vi "UHR-Fleezers Control (fpga) - 11.7.1UCBMeng3RG2.vi"() -> ()   [LabVIEW 2014]
doc: "UHR-Fleezers Instrument Control Code (fpga)"
uses:
  <vilib>/Platform/TimedLoop/XDataNode/timing_clust.ctl
  <vilib>/Platform/TimedLoop/XDataNode/nitl_modes.ctl
  <vilib>/Platform/TimedLoop/XDataNode/wakeup.ctl
  <vilib>/rvi/Emulation/niFpgaGetClockAttributes.vi
  <vilib>/rvi/Emulation/niFpgaSctlEmulationGetInTimedLoop.vi
  <vilib>/rvi/Emulation/niFpgaEmulationReportErrorSimple.vi
  <vilib>/rvi/Emulation/niFpgaProcessEmulError.vi
  <vilib>/rvi/eio/common/nirviEmuTemplateMethod_errors.vi
  <vilib>/rvi/Emulation/niFpgaCriticalErrorInLSC.vi
  <vilib>/rvi/interface/RandomDataEmulation/niFpgaRandomDataHandleErrors.vi
  <vilib>/eio/EIONode/EIONode.xnode
  <vilib>/eio/EIOMethodNode/EIOMethodNode.xnode
  <vilib>/rvi/DataTransferAndStorage/Container/XNode/niFpgaContainer.xnode
  <vilib>/rvi/interface/RandomDataEmulation/nirviRandomDataFpgaReadWriteTemplate.vi
  <vilib>/addons/control/pid/fpga.llb/XNode/niFpgaPID.xnode
  <vilib>/Platform/TimedLoop/XDataNode/XDataNode.xnode
  <vilib>/Platform/TimedLoop/XDataNode/XDNodeRunTimeDep.lvlib
panel:
  in  "Tab Control":T1(tab)=enum."Force FB"
  in  "Set 3":bool
  in  "Set 2":bool=TRUE
  in  "Set 1":bool=TRUE
  in  "Trap Pos to FIFO":bool
  in  "N of AI1 Int Acq Sets":i16=2 min=1 max=3 step=1
  out "AI Late Counter":u8
  in  "ai count":u16=400
  in  "+ phase":bool
  in  "Phase count adjustment":i16
  out "Relative phase":i16
  in  "AI to FIFO":bool
  out "BD1 Frequency Out 1":u64
  out "BD1 Frequency Out 2":u64
  out "Trap Pos FIFO Timeout":u16
  out "Trap AI FIFO Timeout":u16
  in  "Trap FIFO Set Timeout":i32
  in  "Tab Control 2":T2(tab)
  in  "FB Offset":u16
  in  "FB Multi Factor":i16
  in  "Dynamic FB (Ronen)":bool
  in  "Negate Intensity FB":bool
  in  "RD":bool
  in  "FB1 output high":i16=3000
  in  "FB1 output low":i16
  in  "D1":i16
  in  "I1":i16=5
  in  "P1":i16=10
  in  "Swap F1 and F2":bool
  in  "Cont. Scan":bool
  in  "Abort scan":bool
  in  "Cycles per step":u64
  in  "Scan BD":bool
  in  "Number of scans":u16
  in  "Scan steps":u64
  in  "Scan freq.  increment":i64
  out "Scanning":bool
  in  "Start scan":bool
  in  "OSK Bd 1":bool
  in  "Reset Bd 1":bool
  in  "PMODE":bool
  in  "Direct RF Box \nCommunication":bool
  in  "Data BD 2":u8 format="%08b"
  in  "Data BD 1":u8 format="%08b"
  in  "Address":u8 format="%02x"
  in  "Update Data":bool
  in  "FPGA Controls\n RF Box":bool
  in  "Number Interlace Cycles":u8=2 min=1 max=3
  in  "Interlace Off Parameters":u8=1 min=1 max=3
  in  "Interlace ON/OFF":bool
  out "DIO Relative phase":i16
  in  "Phase count adjustment (DIO)":i16
  in  "+ phase (DIO)":bool
  out "DIO Late Counter":u8
  in  "DIO count 1 (ticks)":u16=400
  in  "DIO count 2 (ticks)":u16=400
  in  "DIO count 3 (ticks)":u16=400
  out "AI2 Y Sum Set 2":i16
  out "AI2 Y Sum Set 1":i16
  in  "FB Setpoint Set 1":i16 min=0 step=1
  in  "FB Reset Set 1":bool
  in  "FB On/Off Set 1":bool
  in  "FB Reset Set 2":bool
  in  "FB On/Off Set 2":bool
  in  "FB Setpoint Set 2":i16 min=0 step=1
  out "Scan I":u64
  in  "Amp switch delay":u8=5
  in  "XY phase ext loop method":bool
  in  "BD 2 Amplitude 1":u16
  in  "BD 1 Amplitude 1":u16
  in  "BD 2 Frequency 1":u64
  in  "BD 1 Frequency 1":u64
  in  "BD 2 Amplitude 2":u16
  in  "BD 1 Amplitude 2":u16
  in  "BD 2 Frequency 2":u64
  in  "BD 1 Frequency 2":u64
  in  "BD 2 Amplitude 3":u16
  in  "BD 1 Amplitude 3":u16
  in  "BD 2 Frequency 3":u64
  in  "BD 1 Frequency 3":u64
  in  "BD 1 Delay (ticks)":u8
  in  "BD 2 Delay (Ticks)":u8 caption="Count(Ticks)"
  in  "Next trap write delay (ticks)":u8 caption="Count(Ticks)"
  in  "Trap 1 osc enable":bool
  in  "Trap 2 osc enable":bool
  in  "Dynamic Force FB (Ronen)":bool
  in  "FB2 output high":fxp<+/-,16,1>=0.999969482421875
  in  "FB2 output low":fxp<+/-,16,1>=-1.0
  in  "P2":fxp<+/-,16,8> format="%.11g"
  in  "I2":fxp<+/-,16,8>=10.0 format="%.11g"
  in  "D2":fxp<+/-,16,8> format="%.11g"
  in  "Negate Diff?":bool
  in  "Diff FB Measurement?":bool
  in  "FB Trig Integrate":u32=1
  out "TTrig?":bool
  in  "TTrig Negate Pos":bool=TRUE
  out "Trap Pos FB Int Signal":fxp<+/-,24,9> format="%.18g"
  out "Trap Pos FB Int-Norm Signal":fxp<+/-,16,1> format="%.16g"
  in  "FPGA TTrig Thresh":i64
  in  "FPGA Trap Trig":bool
  out "Trap Pos FB Action":i64
  in  "Trap Pos. FB Offset Factor":i64
  in  "Trap Pos. FB Mult Factor":i64=2
  in  "Trap Pos. FB Reset":bool
  in  "Trap Pos FB Monitor T1 or T2":bool
  in  "AI1 X Scale":u16
  in  "Trap Pos FB Int Count":u16=100
  in  "Trap Pos FB Negate Action":bool
  out "AI1 X Set 2":fxp<+/-,16,1>
  out "AI1 X Set 1":fxp<+/-,16,1>
  in  "Trap Pos. FB SP":fxp<+/-,16,1>
  in  "Force feedback":bool
  out "TTrig Sig":i64
  out "TTrig Fin Thresh":i64
  in  "1D or 2D Scan?":bool
  in  "Abort scan (MCL)":bool
  in  "MCL Scan Axis":bool
  in  "Cont. Scan (MCL)":bool
  out "Scan I (MCL)":u64
  in  "Number of scans (MCL)":u16
  out "Scanning MCL":bool
  in  "Scan steps (MCL)":u64
  in  "Cycles per step (MCL)":u64
  in  "Scan freq.  increment (MCL)":i16
  in  "Start scan (MCL)":bool
  in  "AO2":i16
  in  "AO1":i16
  out "MCL Late Counter":u8
  in  "MCL count":u32=800
  out "MCL Relative Phase":i16
  in  "Phase count adjustment (MCL)":i16
  in  "+ phase (MCL)":bool
  out "APD2 int gate":bool
  out "APD3 out state":bool
  in  "APD Gate Operating Mode":u8 max=2 step=1
  in  "Invert APD Gate":bool
  in  "APD Gate OFF Count":u16=100
  in  "APD Gate ON Count":u16=300
  out "APD 1 Gate Late Counter":u8
  out "APD 1 Gate Relative Phase":i16
  in  "Phase count adjustment (APD 1 Gate)":i16
  in  "+ phase (APD 1 Gate)":bool
  out "APD 2 Counts 0":u32
  out "APD 2 Counts 1":u32
  out "APD 1 Counts 0":u32
  out "APD 1 Counts 1":u32
  out "APD1 out state":bool
  in  "APD AO scale factor":i16=1
  in  "APD to FIFO":bool
  in  "APD Acq Rate Count":u32=20000000
  out "APD Acq Late Counter":u8
  out "APD Acq Relative Phase":i16
  in  "Phase Count Adjustment (APD Acq)":i16
  in  "+ phase (APD Acq)":bool
  in  "Phase count adjustment (APD 2 Gate)":i16
  out "APD 2 Gate Late Counter":u8
  out "APD 2 Gate Relative Phase":i16
  in  "+ phase (APD 2 Gate)":bool
  out "APD2 out state":bool
  out "APD 3 Counts 0":u32
  out "APD 3 Counts 1":u32
  out "APD 3 Gate Late Counter":u8
  in  "Phase count adjustment (APD 3 Gate)":i16
  out "APD 3 Gate Relative Phase":i16
  in  "+ phase (APD 3 Gate)":bool
  out "APD1 int gate":bool
  out "APD3 int gate":bool
  in  "D3":i16
  in  "I3":i16=5
  in  "P3":i16=10
  in  "Green Filter Flipper":bool
  in  "Green FB Count":u16=1200
  out "Green Late Counter":u8
  out "Green FB Relative Phase":i16
  in  "Phase count adjustment (Green FB)":i16=10
  in  "+ phase (Green FB)":bool
  out "Green FB Sum":i16
  in  "Green int current ON count adj":u16=150
  in  "Current Out":u16=30000
  in  "Green FB On/Off":bool
  in  "Green FB Setpoint":i16=250 min=0 step=1
  in  "Green FB Reset":bool
  in  "Operating Mode 2":u8=2 max=2 step=1
  in  "Invert GI 2":bool
  in  "Green interlace OFF count 2":u16=900
  in  "Green interlace ON count 2":u16=300
  out "GI Late Counter 2":u8
  out "GI Relative phase 2":i16
  in  "Phase count adjustment (GI) 2":i16=20
  in  "+ phase (GI) 2":bool
  in  "Green interlace OFF count":u16=100
  out "GI Relative phase":i16
  in  "Phase count adjustment (GI)":i16
  in  "+ phase (GI)":bool
  in  "Green interlace ON count":u16=300
  out "GI Late Counter":u8
  in  "Invert GI":bool
  in  "Operating Mode":u8 max=2 step=1
  in  "+ phase (RI)":bool
  out "RI Relative phase":i16
  out "RI Late Counter":u8
  in  "Red interlace ON count":u16=300
  in  "Red interlace OFF count":u16=100
  in  "Invert RI":bool
  in  "Red Laser Operating Mode":u8 max=2 step=1
  in  "Phase count adjustment (RI)":i16
  out "Red FB Intensity":i16
  in  "RI Current Out":u16=30000
  in  "Red FB On/Off":bool
  in  "D4":i16
  in  "I4":i16=5
  in  "P4":i16=10
  in  "Red FB Setpoint":i16=250 min=0 step=1
  in  "Red FB Reset":bool
  in  "RI Operating Mode 2":u8=2 max=2 step=1
  in  "Invert RI 2":bool
  in  "Phase count adjustment (BI AO)":i16=20
  in  "Blue current ON count adj (AO)":u16=150
  in  "BI Current Out":i16=30000
  in  "Blue FB On/Off":bool
  in  "D5":i16
  in  "I5":i16=5
  in  "P5":i16=10
  in  "Blue FB Setpoint":i16=250 min=0 step=1
  in  "Blue FB Reset":bool
  in  "BI Operating Mode (AO)":u8=2 max=2 step=1
  in  "Invert BI (AO)":bool
  in  "Blue OFF count (AO)":u16=900
  in  "Blue ON count (AO)":u16=300
  out "BI Late Counter (AO)":u8
  out "BI Relative phase (AO)":i16
  in  "+ phase (BI AO)":bool
  in  "Phase count adjustment (BI D)":i16
  in  "Blue Laser Operating Mode (D)":u8 max=2 step=1
  in  "Invert BI (D)":bool
  in  "Blue interlace OFF count (D)":u16=100
  in  "Blue interlace ON count (D)":u16=300
  out "Blue Late Counter (D)":u8
  out "BI Relative phase (D)":i16
  in  "+ phase (BI D)":bool
  out "Blue Intensity":i16
  # "Only one of these can be on\nat a time:"
  # "Raster Scan AOD"
  # "1 (X)"
  # "2 (Y)"
  # "IR Intensity Feedback (RF BD 1)"
  # "FB Gains Set 1"
  # "FB output range 1"
  # "False is usual, True is external loop method"
  # "Parameters if using the external RF switching loop"
  # "Parameters if using the usual internal RF switching method"
  # "FB Triggering Excitation Laser"
  # "Trap Pos. FB Gains"
  # "Trap Pos. FB Range"
  # "AO1 (Y)"
  # "2D"
  # "1D"
  # "AO2 (X)"
  # "APD AO for aligning"
  # "Detection Loop"
  # "Green fluorescent laser digital gate interlacing loop"
  # "0 Forced ON\n1 Forced OFF\n2 Interlacing"
  # "Green FB Gains"
  # "Red fluorescent laser digital gate interlacing loop"
  # "Detection Loop"
  # "0 Forced ON\n1 Forced OFF\n2 Interlacing"
  # "Analog/FB Control Loop\n(Disabled)"
  # "Digital Control Loop"
  # "Blue laser intensity reading"
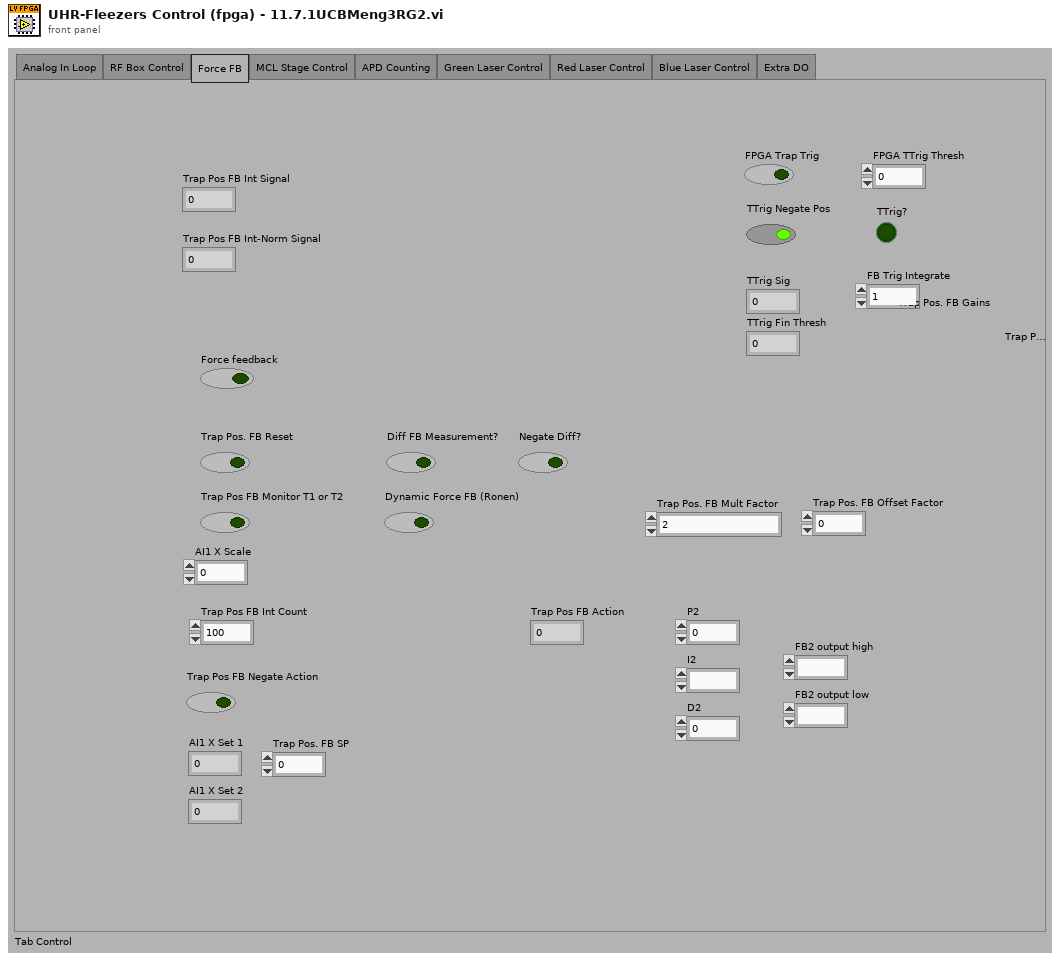
[diagram p1: front panel]
types:
  T1 = enum32{"Analog In Loop", "RF Box Control", "Force FB", "MCL Stage Control", "APD Counting", "Green Laser Control", "Red Laser Control", "Blue Laser Control", "Extra DO"}
  T2 = enum32{"Controls", "Interlacing Frequency and Amplitude Values", "Oscillate trap from memory"}
  T3 = typedef "XDNodeRunTimeDep.lvlib/timing_clust.ctl" = cluster{"Expected End [f-1]":u64, "Actual End [f-1]":u64, "Finished Late? [f-1]":bool, "Expected End [i-1]":u64, "Actual End [i-1]":u64, "Finished Late? [i-1]":bool, "Expected Start [i]":u64, "Actual Start [i]":u64, "Expected Start [f]":u64, "Actual Start [f]":u64, "Source Name":string, "Structure Name":string, "Period":i64, "Deadline":i64, "Offset":i64, "Start":i64, "Priority":i32, "Timeout":i32, "Mode":T4, "Wakeup Reason":T5, "Error":errorcluster, "Source Type":string, "Secondary Source Type":string, "Global End Time":u64, "Global Start Time":u64, "Frame Duration":u64, "Iteration Duration":u64, "Assigned CPU":i32, "I/O Scan Engine Mode":u32}
  T4 = typedef "XDNodeRunTimeDep.lvlib/nitl_modes.ctl" = enum32{"No Change", "Process missed periods, maintain original phase", "Discard missed periods, maintain original phase", "Process missed periods, ignore original phase", "Discard missed periods, ignore original phase"}
  T5 = typedef "XDNodeRunTimeDep.lvlib/wakeup.ctl" = enum32{"Normal", "Aborted", "Asynchronous wakeup", "Timing source error", "Timed loop error", "Timeout"}
  T6 = cluster{"proportional gain (Kc)":i16, "integral gain (Kc*Ts/Ti)":i16, "derivative gain (Kc*Td/Ts)":i16}
  T7 = cluster{"FB1 output high":i16, "FB1 output low":i16}
  T8 = cluster{"P2":fxp<+/-,16,8>, "I2":fxp<+/-,16,8>, "D2":fxp<+/-,16,8>}
  T9 = cluster{"FB2 output high":fxp<+/-,16,1>, "FB2 output low":fxp<+/-,16,1>}
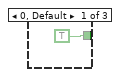
[diagram p2: hidden frame]
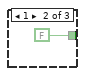
[diagram p3: hidden frame]
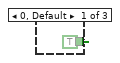
[diagram p4: hidden frame]
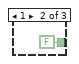
[diagram p5: hidden frame]
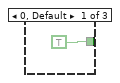
[diagram p7: hidden frame]
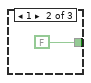
[diagram p8: hidden frame]
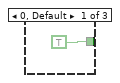
[diagram p10: hidden frame]
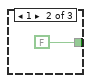
[diagram p11: hidden frame]
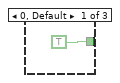
[diagram p14: hidden frame]
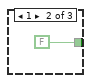
[diagram p15: hidden frame]
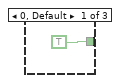
[diagram p17: hidden frame]
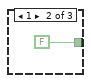
[diagram p18: hidden frame]
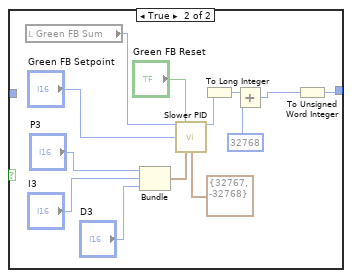
[diagram p20: hidden frame]
diagram:
  w7 = FALSE
  w5 = FALSE
  # "timing array current index"
  # "timing array"
  # "timing counter (phase adjusted here)"
  # "late counter"
  n1 = flat-sequence "FPGA initialization to do before running any of the loops" {
    tunnel: [u16 0 ("DIO count 3 (ticks)")] -> w4
    tunnel: [w15] -> _
    frame #0 {
      w14 = FALSE ("Enable")
      # "BD 2 (Y)"
      # "BD 1 (X)"
      # "Start up expansion chassis early\nto avoid delays later"
      # "This pin controls udclk on the RF boards.\nWhen initially configuring the boards, this pin needs to be\nconfigured as a high impedance input.  Later it will be switched\nto an output."
      # "Initial setting of DIO data and \naddress to low (before reset).  \nThis needs to happen before the other\ncontrol method loops execute."
      n2 = xnode "FPGA I/O Node"("Chassis2/Mod1/AO0"=u16 0 ("Chassis2/Mod4/AO0")) -> ("Chassis2/Mod2/AI0"=w15:i16)  [unwired: 2 in, 2 out]
      n3 = xnode "FPGA I/O Method Node"("Enable"=w14) -> ()  [unwired: 1 in, 1 out]
      n4 = xnode "FPGA I/O Method Node"("Enable"=w14) -> ()  [unwired: 1 in, 1 out]
      n5 = xnode "FPGA I/O Node"("Connector1/DIO0"=FALSE, "Connector1/DIO1"=FALSE, "Connector1/DIO2"=FALSE, "Connector1/DIO3"=FALSE, "Connector1/DIO4"=FALSE, "Connector1/DIO5"=FALSE, "Connector1/DIO6"=FALSE, "Connector1/DIO7"=FALSE, "Connector1/DIO8"=FALSE, "Connector1/DIO9"=FALSE, "Connector1/DIO10"=FALSE, "Connector1/DIO11"=FALSE, "Connector1/DIO12"=FALSE, "Connector1/DIO13"=FALSE, "Connector1/DIO15"=FALSE, "Connector1/DIO20"=FALSE, "Connector1/DIO21"=FALSE, "Connector1/DIO22"=FALSE, "Connector1/DIO23"=FALSE, "Connector1/DIO24"=FALSE, "Connector1/DIO25"=FALSE, "Connector1/DIO26"=FALSE, "Connector1/DIO27"=FALSE, "Connector1/DIO14"=FALSE) -> ()  [unwired: 24 in, 24 out]
    }
  }
  n6 = local read "AO1"() -> (w12:i16)
  n7 = local read "AO2"() -> (w11:i16)
  n8 = node-c288() -> (w10:T3)  [unwired: 1 in]
  n9 = To Unsigned Long Integer(number=w4) -> (unsigned 32bit integer=w8:u32)
  n10 = timed-loop "RF box board DIO control: control bits" {
    timing: w10 -> [_]
    timing-out: [_] -> w9
    tunnel: [w44] -> _
    tunnel: w4 -> [w44]
    stop <- FALSE stop-if-true
    n11 = xnode "FPGA I/O Node"("Connector1/DIO16"="RD", "Connector1/DIO17"="PMODE", "Connector1/DIO18"="OSK Bd 1", "Connector1/DIO19"="Reset Bd 1", "Connector0/DIO3"="Green Filter Flipper") -> ()  [unwired: 5 in, 5 out]
  }
  n12 = disable-structure shown="Disabled" {
    disable-tunnel: w7 -> [w52 _]
    disable-tunnel: w4 -> [w51 _]
    frame Disabled {
      n13 = while "APD 2 Gating" {
        shift-right: [w56] -> _
        shift-left: w51 -> [w61]
        shift-right: [w55] -> _
        shift-left: w52 -> [w53]
        stop <- FALSE stop-if-true
        n14 = flat-sequence {
          tunnel: w61 -> [w64]
          tunnel: [w65] -> w59
          tunnel: [w64] -> w57
          tunnel: [w63] -> w54
          tunnel: w53 -> [w63]
          tunnel: [w68] -> w60
          tunnel: w59 -> [w68]
          tunnel: [w67] -> w58
          tunnel: w57 -> [w67]
          tunnel: w54 -> [w66]
          tunnel: [w90] -> w56
          tunnel: w60 -> [w100]
          tunnel: w58 -> [w98]
          tunnel: [w69] -> w55
          frame #0 {
            n15 = call "Loop Timer8"("Count(Ticks)"=w64) -> ("Tick Count(Ticks)"=w65:u16)
          }
          frame #1 {
            # "Signal maybe then sent through \na transistor before APD"
            n16 = xnode "FPGA I/O Node"("Connector0/DIO8"=w66, "Connector0/DIO9"=w66, "Connector0/DIO10"=w66, "Connector0/DIO11"=w66) -> ()  [unwired: 4 in, 4 out]
            "APD2 int gate" <- w66
          }
          frame #2 {
            n17 = local read "APD Gate ON Count"() -> (w83:u16)
            n18 = local read "APD Gate OFF Count"() -> (w82:u16)
            n19 = feedback #1(TRUE) -> (w95:bool)
            n20 = feedback-in #2(w100) -> ()
            n21 = feedback #2(w100) -> (w84:u16)
            n22 = Not(x=w95) -> (.not. x?=w93:bool)
            n23 = feedback-in #1(w93) -> ()
            n24 = Subtract(x=w100, y=w84) -> (x-y=w99:u16)
            n25 = Select(t=w83, s=w93, f=w82) -> (s? t:f=w97:u16)
            n26 = Subtract(x=w99, y=w98) -> (x-y=w75:u16)
            n27 = Subtract(x=w97, y=w75) -> (x-y=w89:u16)
            n28 = Number To Boolean Array(number=w75) -> (Boolean array=w74:bool[])
            n29 = Or Array Elements(Boolean array=w74) -> (logical OR=w73:bool)
            n30 = Boolean To (0,1)(Boolean="+ phase (APD 2 Gate)") -> (0, 1=w87:i16)
            n31 = Multiply(x=w87, y="Phase count adjustment (APD 2 Gate)") -> (x*y=w85:i16)
            n32 = Boolean To (0,1)(Boolean=w73) -> (0, 1=w80:i16)
            n33 = Add(x=w89, y=w85) -> (x+y=w90:u16)
            n34 = To Unsigned Byte Integer(number=w80) -> (unsigned 8bit integer=w77:u8)
            n35 = feedback #3(i16 0) -> (w92:i16)
            n36 = Subtract(x=w92, y=w85) -> (x-y=w91:i16)
            "APD 2 Gate Relative Phase" <- w91
            n37 = feedback-in #3(w91) -> ()
            n38 = feedback #4(u8 0) -> (w78:u8)
            n39 = Add(x=w77, y=w78) -> (x+y=w76:u8)
            "APD 2 Gate Late Counter" <- w76
            n40 = feedback-in #4(w76) -> ()
            n41 = local read "APD Gate Operating Mode"() -> (w81:u8)
            n42 = case shown="2" w81 {
              tunnel: [TRUE FALSE w103] -> w70
              tunnel: w95 -> [_ _ w103]
              frame 0, Default {
              }
              frame 1 {
              }
              frame 2 {
              }
            }
            n43 = local read "Invert APD Gate"() -> (w72:bool)
            n44 = Not(x=w70) -> (.not. x?=w71:bool)
            n45 = Select(t=w71, s=w72, f=w70) -> (s? t:f=w69:bool)
          }
        }
      }
      n46 = while "APD 1 Gating" {
        shift-right: [w107] -> _
        shift-left: w51 -> [w112]
        shift-right: [w106] -> _
        shift-left: w52 -> [w104]
        stop <- FALSE stop-if-true
        n47 = flat-sequence {
          tunnel: w112 -> [w115]
          tunnel: [w116] -> w110
          tunnel: [w115] -> w108
          tunnel: [w114] -> w105
          tunnel: w104 -> [w114]
          tunnel: [w119] -> w111
          tunnel: w110 -> [w119]
          tunnel: [w118] -> w109
          tunnel: w108 -> [w118]
          tunnel: w105 -> [w117]
          tunnel: [w137] -> w107
          tunnel: w111 -> [w151]
          tunnel: w109 -> [w148]
          tunnel: [w120] -> w106
          frame #0 {
            n48 = call "Loop Timer7"("Count(Ticks)"=w115) -> ("Tick Count(Ticks)"=w116:u16)
          }
          frame #1 {
            # "Signal maybe then sent through \na transistor before APD"
            n49 = xnode "FPGA I/O Node"("Connector0/DIO4"=w117, "Connector0/DIO5"=w117, "Connector0/DIO6"=w117, "Connector0/DIO7"=w117) -> ()  [unwired: 4 in, 4 out]
            "APD1 int gate" <- w117
          }
          frame #2 {
            n50 = feedback #5(TRUE) -> (w143:bool)
            n51 = feedback-in #6(w151) -> ()
            n52 = feedback #6(w151) -> (w150:u16)
            n53 = Not(x=w143) -> (.not. x?=w140:bool)
            n54 = feedback-in #5(w140) -> ()
            n55 = Subtract(x=w151, y=w150) -> (x-y=w149:u16)
            n56 = Select(t="APD Gate ON Count", s=w140, f="APD Gate OFF Count") -> (s? t:f=w145:u16)
            n57 = Subtract(x=w149, y=w148) -> (x-y=w125:u16)
            n58 = Subtract(x=w145, y=w125) -> (x-y=w136:u16)
            n59 = Number To Boolean Array(number=w125) -> (Boolean array=w126:bool[])
            n60 = Or Array Elements(Boolean array=w126) -> (logical OR=w124:bool)
            n61 = Boolean To (0,1)(Boolean="+ phase (APD 1 Gate)") -> (0, 1=w134:i16)
            n62 = Boolean To (0,1)(Boolean=w124) -> (0, 1=w131:i16)
            n63 = Multiply(x=w134, y="Phase count adjustment (APD 1 Gate)") -> (x*y=w132:i16)
            n64 = To Unsigned Byte Integer(number=w131) -> (unsigned 8bit integer=w128:u8)
            n65 = Add(x=w136, y=w132) -> (x+y=w137:u16)
            n66 = feedback #7(i16 0) -> (w139:i16)
            n67 = Subtract(x=w139, y=w132) -> (x-y=w138:i16)
            "APD 1 Gate Relative Phase" <- w138
            n68 = feedback-in #7(w138) -> ()
            n69 = feedback #8(u8 0) -> (w129:u8)
            n70 = Add(x=w128, y=w129) -> (x+y=w127:u8)
            "APD 1 Gate Late Counter" <- w127
            n71 = feedback-in #8(w127) -> ()
            n72 = case shown="2" "APD Gate Operating Mode" {
              tunnel: [TRUE FALSE w154] -> w121
              tunnel: w143 -> [_ _ w154]
              frame 0, Default {
              }
              frame 1 {
              }
              frame 2 {
              }
            }
            n73 = Not(x=w121) -> (.not. x?=w122:bool)
            n74 = Select(t=w122, s="Invert APD Gate", f=w121) -> (s? t:f=w120:bool)
          }
        }
      }
    }
    frame Enabled {
    }
  }
  n75 = while "RF box board direct communication loop" {
    tunnel: w4 -> [_]
    stop <- FALSE stop-if-true
    n76 = case "Whether to use direct communication method (only use one method at a time)" shown="True" "Direct RF Box \nCommunication" {
      frame False {
      }
      frame True {
        n77 = case shown="True" "Update Data" {
          frame False {
          }
          frame True {
            n78 = flat-sequence {
              frame #0 {
                n79 = First Call?() -> (First Call?: T/F=w158:bool)
                n80 = case shown="True" w158 {
                  frame False {
                  }
                  frame True {
                    # "If first time data updated, be sure to set WR high\nbefore setting data and address bits."
                    n81 = flat-sequence {
                      frame #0 {
                        n82 = xnode "FPGA I/O Node"("Connector1/DIO15"=TRUE) -> ()  [unwired: 1 in, 1 out]
                      }
                      frame #1 {
                        n83 = call "Wait"("Count(Ticks)"=u8 40 ("DO Delay 3 (Ticks)")) -> ()  [unwired: 1 out]
                      }
                    }
                  }
                }
              }
              frame #1 {
                n84 = Number To Boolean Array(number="Address") -> (Boolean array=w207:bool[])
                n85 = Number To Boolean Array(number="Data BD 1") -> (Boolean array=w208:bool[])
                n86 = Number To Boolean Array(number="Data BD 2") -> (Boolean array=w177:bool[])
                n87 = Index Array(array=w208, index=7) -> (element=w192:bool)
                n88 = Index Array(array=w208, index=6) -> (element=w191:bool)
                n89 = Index Array(array=w208, index=5) -> (element=w190:bool)
                n90 = Index Array(array=w208, index=4) -> (element=w189:bool)
                n91 = Index Array(array=w208, index=3) -> (element=w188:bool)
                n92 = Index Array(array=w208, index=2) -> (element=w187:bool)
                n93 = Index Array(array=w208, index=1) -> (element=w186:bool)
                n94 = Index Array(array=w208, index=0) -> (element=w185:bool)
                n95 = Index Array(array=w207, index=5) -> (element=w184:bool)
                n96 = Index Array(array=w207, index=4) -> (element=w183:bool)
                n97 = Index Array(array=w207, index=3) -> (element=w182:bool)
                n98 = Index Array(array=w207, index=2) -> (element=w181:bool)
                n99 = Index Array(array=w207, index=1) -> (element=w180:bool)
                n100 = Index Array(array=w207, index=0) -> (element=w179:bool)
                n101 = Index Array(array=w177, index=7) -> (element=w168:bool)
                n102 = Index Array(array=w177, index=6) -> (element=w167:bool)
                n103 = Index Array(array=w177, index=5) -> (element=w166:bool)
                n104 = Index Array(array=w177, index=4) -> (element=w165:bool)
                n105 = Index Array(array=w177, index=3) -> (element=w164:bool)
                n106 = Index Array(array=w177, index=2) -> (element=w163:bool)
                n107 = Index Array(array=w177, index=1) -> (element=w162:bool)
                n108 = Index Array(array=w177, index=0) -> (element=w161:bool)
                n109 = xnode "FPGA I/O Node"("Connector1/DIO0"=w192, "Connector1/DIO1"=w191, "Connector1/DIO2"=w190, "Connector1/DIO3"=w189, "Connector1/DIO4"=w188, "Connector1/DIO5"=w187, "Connector1/DIO6"=w186, "Connector1/DIO7"=w185, "Connector1/DIO8"=w184, "Connector1/DIO9"=w183, "Connector1/DIO10"=w182, "Connector1/DIO11"=w181, "Connector1/DIO12"=w180, "Connector1/DIO13"=w179, "Connector1/DIO20"=w168, "Connector1/DIO21"=w167, "Connector1/DIO22"=w166, "Connector1/DIO23"=w165, "Connector1/DIO24"=w164, "Connector1/DIO25"=w163, "Connector1/DIO26"=w162, "Connector1/DIO27"=w161) -> ()  [unwired: 22 in, 22 out]
              }
              frame #2 {
                # "wait and then apply write signal"
                n110 = call "Wait2"("Count(Ticks)"=u8 40 ("DO Delay 1 (Ticks)")) -> ()  [unwired: 1 out]
              }
              frame #3 {
                # "sending bit low writes data to board buffer"
                n111 = xnode "FPGA I/O Node"("Connector1/DIO15"=FALSE) -> ()  [unwired: 1 in, 1 out]
              }
              frame #4 {
                # "wait then return write signal"
                n112 = call "Wait3"("Count(Ticks)"=u8 40 ("DO Delay 2 (Ticks)")) -> ()  [unwired: 1 out]
              }
              frame #5 {
                # "sending bit high makes ready to\nwrite more data"
                n113 = xnode "FPGA I/O Node"("Connector1/DIO15"=TRUE) -> ()  [unwired: 1 in, 1 out]
              }
            }
          }
        }
      }
    }
  }
  n114 = while "RF box board DIO control: parallel communication" {
    shift-right: [w227] -> _
    shift-left: w4 -> [w226]
    shift-right: [w225] -> _
    shift-left: FALSE ("Swap F1 and F2") -> [w224]
    shift-right: [w219] -> _
    shift-left: u16 0 -> [w220]
    shift-right: [w217] -> _
    shift-left: u16 0 -> [w218]
    shift-right: [w215] -> _
    shift-left: u64 0 -> [w216]
    stop <- FALSE stop-if-true
    n115 = flat-sequence {
      tunnel: w224 -> [w231]
      tunnel: w226 -> [w229]
      tunnel: [w231] -> w223
      tunnel: [w230] -> w222
      tunnel: [w229] -> w221
      tunnel: [w243] -> w227
      tunnel: [w242] -> w225
      tunnel: w223 -> [w241]
      tunnel: w222 -> [w239]
      tunnel: w221 -> [w238]
      tunnel: w220 -> [w237]
      tunnel: [w236] -> w219
      tunnel: w218 -> [w235]
      tunnel: [w234] -> w217
      tunnel: w216 -> [w233]
      tunnel: [w232] -> w215
      frame #0 {
        n116 = call "Loop Timer"("Count(Ticks)"=w229) -> ("Tick Count(Ticks)"=w230:u16)
      }
      frame #1 {
        n117 = flat-sequence {
          tunnel: ["FPGA Controls\n RF Box"] -> w240
          tunnel: w241 -> [w244]
          tunnel: [w307] -> w243
          tunnel: [w320] -> w242
          tunnel: w240 -> [w319]
          tunnel: w239 -> [w313]
          tunnel: w238 -> [w310]
          tunnel: w237 -> [w276]
          tunnel: [w275] -> w236
          tunnel: w235 -> [w272]
          tunnel: [w271] -> w234
          tunnel: w233 -> [w270]
          tunnel: [w269] -> w232
          frame #0 {
            n118 = case shown="True" "FPGA Controls\n RF Box" {
              tunnel: w244 -> [_ w246]
              frame False {
              }
              frame True {
                n119 = flat-sequence {
                  tunnel: w246 -> [w256]
                  frame #0 {
                    n120 = First Call?() -> (First Call?: T/F=w247:bool)
                    n121 = case shown="True" w247 {
                      frame False {
                      }
                      frame True {
                        # "BD 2"
                        # "BD 1"
                        # "If first time data updated, be sure to set WR high and UDCLK low\nbefore setting data and address bits."
                        n122 = xnode "FPGA I/O Method Node"("Enable"=TRUE) -> ("FPGA I/O Out"=w249:refnum<k21>)  [unwired: 1 in]
                        n123 = xnode "FPGA I/O Method Node"("Enable"=TRUE) -> ("FPGA I/O Out"=w252:refnum<k21>)  [unwired: 1 in]
                        n124 = xnode "FPGA I/O Node"("Connector1/DIO15"=TRUE) -> ()  [unwired: 1 in, 1 out]
                        n125 = xnode "FPGA I/O Node"("I/O Item"=FALSE ("Connector1/DIO30"), "FPGA I/O In"=w249) -> ()  [unwired: 1 out]
                        n126 = xnode "FPGA I/O Node"("I/O Item"=FALSE ("Connector1/DIO30"), "FPGA I/O In"=w252) -> ()  [unwired: 1 out]
                      }
                    }
                  }
                  frame #1 {
                    n127 = case shown="False" FALSE {
                      tunnel: w256 -> [w258 _]
                      frame False {
                        # "Usual operation"
                        n128 = flat-sequence "BD 1 (X)" {
                          tunnel: w258 -> [w265]
                          tunnel: "Amp switch delay" -> [w266]
                          frame #0 {
                            n129 = call "Wait6"("Count(Ticks)"="BD 1 Delay (ticks)") -> ()  [unwired: 1 out]
                          }
                          frame #1 {
                            # "switch frequency"
                            n130 = xnode "FPGA I/O Node"("Connector1/DIO36"=w265) -> ()  [unwired: 1 in, 1 out]
                          }
                          frame #2 {
                            # "~5 ticks is usual"
                            n131 = call "Wait4"("Count(Ticks)"=w266) -> ()  [unwired: 1 out]
                          }
                          frame #3 {
                            # "this switches amplitude"
                            # "switch amplitude"
                            # "send udclk high"
                            n132 = xnode "FPGA I/O Node"("Connector1/DIO30"=TRUE ("Connector1/DIO15")) -> ()  [unwired: 1 in, 1 out]
                          }
                          frame #4 {
                            # "reset to be ready for next\ncycle"
                            # "send udclk low"
                            n133 = xnode "FPGA I/O Node"("Connector1/DIO30"=FALSE ("Connector1/DIO15")) -> ()  [unwired: 1 in, 1 out]
                          }
                        }
                        n134 = flat-sequence "BD 2 (Y)" {
                          tunnel: w258 -> [w260]
                          tunnel: "Amp switch delay" -> [w261]
                          frame #0 {
                            n135 = call "Wait7"("Count(Ticks)"="BD 2 Delay (Ticks)") -> ()  [unwired: 1 out]
                          }
                          frame #1 {
                            # "switch frequency"
                            n136 = xnode "FPGA I/O Node"("Connector1/DIO37"=w260) -> ()  [unwired: 1 in, 1 out]
                          }
                          frame #2 {
                            # "~5 ticks is usual"
                            n137 = call "Wait5"("Count(Ticks)"=w261) -> ()  [unwired: 1 out]
                          }
                          frame #3 {
                            # "this switches amplitude"
                            # "switch amplitude"
                            # "send udclk high"
                            n138 = xnode "FPGA I/O Node"("Connector1/DIO29"=TRUE ("Connector1/DIO15")) -> ()  [unwired: 1 in, 1 out]
                          }
                          frame #4 {
                            # "reset to be ready for next\ncycle"
                            # "send udclk low"
                            n139 = xnode "FPGA I/O Node"("Connector1/DIO29"=FALSE ("Connector1/DIO15")) -> ()  [unwired: 1 in, 1 out]
                          }
                        }
                      }
                      frame True {
                        # "Operation when you need a long delay for either X or Y to synchonize AOD light out phase (> ~100 ticks)."
                        # "Trigger the external loop by sending the boolean FSK value through a FIFO"
                      }
                    }
                  }
                }
              }
            }
          }
          frame #1 {
            # "This is the prior cycle's on time"
            # "increment timing\nindex, reset to 0 if \nend of matrix"
            # "Reset to begginning (1) when number of cycles reached."
            # "timing index"
            # "build byte stacks for writing data\n(must correspond to addresses array constant)"
            # "Timing housekeeping"
            # "Adjust phase if late\n(maintains constant phase relationship between cycles)"
            n140 = Bundle("FB1 output high"="FB1 output high", "FB1 output low"="FB1 output low") -> (w280:T7)  [unwired: 1 in]
            n141 = Bundle("P1"="P1", "I1"="I1", "D1"="D1") -> (w281:cluster{"P1":i16, "I1":i16, "D1":i16})  [unwired: 1 in]
            n142 = feedback #9(u8 0 ("t")) -> (w316:u8)
            n143 = Increment(x=w316) -> (x+1=w359:u8)
            n144 = Increment(x="Number Interlace Cycles") -> (x+1=w354:u8)
            n145 = Equal?(x=w359, y=w354) -> (x = y?=w361:bool)
            n146 = Select(t=u8 1, s=w361, f=w359) -> (s? t:f=w315:u8)
            n147 = feedback-in #9(w315) -> ()
            n148 = Increment(x=w315) -> (x+1=w356:u8)
            n149 = Equal?(x=w356, y=w354) -> (x = y?=w357:bool)
            n150 = Select(t=u8 1, s=w357, f=w356) -> (s? t:f=w353:u8)
            n151 = Select(t=w353, s="Interlace ON/OFF", f="Interlace Off Parameters") -> (s? t:f=w279:u8)
            n152 = case shown="2" w279 {
              tunnel: [w401 w652 "BD 1 Frequency 3"] -> w349
              tunnel: [w447 "BD 2 Frequency 2" "BD 2 Frequency 3"] -> w338
              tunnel: ["BD 2 Amplitude 1" "BD 2 Amplitude 2" "BD 2 Amplitude 3"] -> w295
              tunnel: [w406 w646 "BD 1 Amplitude 3"] -> w298
              tunnel: w281 -> [w414 w654 _]
              tunnel: w280 -> [w415 w653 _]
              tunnel: "Negate Intensity FB" -> [w413 w650 _]
              tunnel: "Dynamic FB (Ronen)" -> [w412 w649 _]
              tunnel: w276 -> [w407 w648 w700]
              tunnel: [w406 w648 w700] -> w275
              tunnel: "FB Multi Factor" -> [w405 w645 _]
              tunnel: "FB Offset" -> [w404 w644 _]
              tunnel: w272 -> [w403 w647 w699]
              tunnel: [w403 w646 w699] -> w271
              tunnel: w270 -> [w402 w643 w698]
              tunnel: [w401 w643 w698] -> w269
              frame 1, Default {
                w430 = fxp<+/-,24,9> 0.0 ("AI1 X Set 2")
                w423 = u16 0
                w443 = u64 0 ("f")
                # "Changed by Ronen - correction \nby PID is now implemented not on \nthe Base BD1 frequency but on the last\nfrequency sent."
                # "BD1 Amp 1"
                # "Changed by Ronen-\n FB changed \nso that value from PID is added to\nlast amplitude sent to board. Correction\nValue can be scaled down same as the force\nFB value."
                # "This signal integration happens no matter what\nso that correct setpoints can be chosen before \nturning on the FB."
                # "Trap 1"
                n153 = local read "AI1 X Set 2"() -> (w426:fxp<+/-,16,1>)
                n154 = local read "AI1 X Set 1"() -> (w427:fxp<+/-,16,1>)
                n155 = local read "Scanning"() -> (w448:bool)
                n156 = Or(x=w448, y="Start scan") -> (x .or. y?=w441:bool)
                n157 = case shown="True" "Diff FB Measurement?" {
                  tunnel: w426 -> [w466 w475]
                  tunnel: w427 -> [w465 w476]
                  tunnel: [w463 w467] -> w428
                  frame False {
                    n158 = Select(t=w465, s="Trap Pos FB Monitor T1 or T2", f=w466) -> (s? t:f=w463:fxp<+/-,16,1>)
                  }
                  frame True {
                    n159 = Subtract(x=w476, y=w475) -> (x-y=w468:fxp<+/-,17,2>)
                    n160 = Not(x="Negate Diff?") -> (.not. x?=w474:bool)
                    n161 = Boolean To (0,1)(Boolean="Negate Diff?") -> (0, 1=w472:i16)
                    n162 = Boolean To (0,1)(Boolean=w474) -> (0, 1=w473:i16)
                    n163 = Negate(x=w472) -> (-x=w471:i16)
                    n164 = Add(x=w471, y=w473) -> (x+y=w469:i16)
                    n165 = Multiply(x=w469, y=w468) -> (x*y=w467:fxp<+/-,32,17>)
                  }
                }
                n166 = Not(x="Abort scan") -> (.not. x?=w439:bool)
                n167 = And(x=w439, y=w441) -> (x .and. y?=w438:bool)
                n168 = case "For raster scanning" shown="False" w438 {
                  tunnel: [u64 0 w602] -> w444
                  tunnel: "Start scan" -> [_ w587]
                  frame False {
                    n169 = local write "Scanning"(FALSE ("scanning")) -> ()
                  }
                  frame True {
                    w571 = i64 0
                    w570 = u64 0
                    # "scan incr."
                    # "freq. incr. mult."
                    # "count steps"
                    # "count number of cycles"
                    n170 = feedback #10(w570) -> (w599:u64)
                    n171 = Select(t=w570, s=w587, f=w599) -> (s? t:f=w601:u64)
                    n172 = Increment(x=w601) -> (x+1=w598:u64)
                    n173 = Greater?(x="Cycles per step", y=w598) -> (0:w580:bool)
                    n174 = Select(t=w598, s=w580, f=w570) -> (s? t:f=w597:u64)
                    n175 = feedback-in #10(w597) -> ()
                    n176 = feedback #11(w570) -> (w596:u64)
                    n177 = Select(t=w570, s=w587, f=w596) -> (s? t:f=w591:u64)
                    n178 = Increment(x=w591) -> (x+1=w595:u64)
                    n179 = Add(x="Scan steps", y="Scan steps") -> (x+y=w594:u64)
                    n180 = Select(t=w591, s=w580, f=w595) -> (s? t:f=w575:u64)
                    n181 = Greater?(x=w594, y=w575) -> (0:w574:bool)
                    n182 = Select(t=w575, s=w574, f=w570) -> (s? t:f=w592:u64)
                    n183 = feedback-in #11(w592) -> ()
                    n184 = Equal?(x="Scan steps", y=w575) -> (x = y?=w579:bool)
                    n185 = Greater?(x="Scan steps", y=w591) -> (0:w590:bool)
                    n186 = feedback #12(w571) -> (w593:i64)
                    n187 = Select(t=w571, s=w587, f=w593) -> (s? t:f=w577:i64)
                    n188 = Increment(x=w577) -> (x+1=w589:i64)
                    n189 = Decrement(x=w577) -> (x-1=w588:i64)
                    n190 = Select(t=w589, s=w590, f=w588) -> (s? t:f=w578:i64)
                    n191 = Select(t=w577, s=w579, f=w578) -> (s? t:f=w576:i64)
                    n192 = Select(t=w577, s=w580, f=w576) -> (s? t:f=w572:i64)
                    n193 = Select(t=w572, s=w574, f=w571) -> (s? t:f=w573:i64)
                    n194 = feedback-in #12(w573) -> ()
                    n195 = feedback #13(w570) -> (w586:u64)
                    n196 = Select(t=w570, s=w587, f=w586) -> (s? t:f=w582:u64)
                    n197 = Increment(x=w582) -> (x+1=w583:u64)
                    n198 = Select(t=w582, s=w574, f=w583) -> (s? t:f=w581:u64)
                    n199 = Greater?(x="Number of scans", y=w581) -> (0:w567:bool)
                    n200 = Multiply(x="Scan freq.  increment", y=w577) -> (x*y=w602:i64)
                    n201 = Select(t=TRUE, s="Cont. Scan", f=w567) -> (s? t:f=w566:bool)
                    "Scanning" <- w566
                    n202 = Select(t=w581, s=w566, f=w570) -> (s? t:f=w584:u64)
                    n203 = feedback-in #13(w584) -> ()
                    n204 = Increment(x=w581) -> (x+1=→"Scan I":u64)
                  }
                }
                n205 = feedback #14(w423) -> (w422:u16)
                n206 = Increment(x=w422) -> (x+1=w424:u16)
                n207 = Greater Or Equal?(x=w424, y="Trap Pos FB Int Count") -> (x >= y?=w400:bool)
                n208 = Select(t=w423, s=w400, f=w424) -> (s? t:f=w425:u16)
                n209 = feedback-in #14(w425) -> ()
                n210 = feedback #15(w430) -> (w429:fxp<+/-,24,9>)
                n211 = Add(x=w428, y=w429) -> (x+y=w421:fxp<+/-,24,9>)
                n212 = case "For intensity feedback" shown="True" "FB On/Off Set 1" {
                  tunnel: w407 -> [_ w607]
                  tunnel: ["BD 1 Amplitude 1" w613] -> w406
                  tunnel: w415 -> [_ w614]
                  tunnel: w414 -> [_ w615]
                  tunnel: w413 -> [_ w612]
                  tunnel: w412 -> [_ w611]
                  tunnel: w405 -> [_ w606]
                  tunnel: w404 -> [_ w605]
                  frame False {
                  }
                  frame True {
                    n213 = local read "AI2 Y Sum Set 1"() -> (w609:i16)
                    n214 = case shown="True" w611 {
                      tunnel: w615 -> [w621 w635]
                      tunnel: w614 -> [w622 w634]
                      tunnel: [w616 w633] -> w613
                      tunnel: w612 -> [_ w632]
                      tunnel: "FB Setpoint Set 1" -> [w620 w631]
                      tunnel: w609 -> [w619 w630]
                      tunnel: "FB Reset Set 1" -> [w618 w629]
                      tunnel: w607 -> [_ w628]
                      tunnel: w606 -> [_ w626]
                      tunnel: w605 -> [_ w624]
                      frame False {
                        n215 = call "Slower PID.vi"("process variable"=w619, "reset?"=w618, "setpoint"=w620, "PID gains (x 2^8)"=w621, "output range"=w622) -> ("output"=w617:i16)  [unwired: 10 out]
                        n216 = To Unsigned Word Integer(number=w617) -> (unsigned 16bit integer=w616:u16)
                      }
                      frame True {
                        n217 = call "Slower PID.vi"("process variable"=w630, "reset?"=w629, "setpoint"=w631, "PID gains (x 2^8)"=w635, "output range"=w634) -> ("output"=w636:i16)  [unwired: 10 out]
                        n218 = To Unsigned Word Integer(number=w636) -> (unsigned 16bit integer=w627:u16)
                        n219 = Scale By Power Of 2(n=w626, x=w627) -> (x*2^n=w625:u16)
                        n220 = Add(x=w625, y=w624) -> (x+y=w623:u16)
                        n221 = case shown="True" w632 {
                          tunnel: w623 -> [w639 w641]
                          tunnel: w628 -> [w637 w642]
                          tunnel: [w638 w640] -> w633
                          frame False {
                            n222 = Add(x=w637, y=w639) -> (x+y=w638:u16)
                          }
                          frame True {
                            n223 = Subtract(x=w642, y=w641) -> (x-y=w640:u16)
                          }
                        }
                      }
                    }
                  }
                }
                n224 = Select(t=w430, s=w400, f=w421) -> (s? t:f=w433:fxp<+/-,24,9>)
                n225 = feedback-in #15(w433) -> ()
                n226 = Divide(x=w421, y="Trap Pos FB Int Count") -> (x/y=w416:fxp<+/-,16,1>)
                n227 = feedback #16(fxp<+/-,24,9> 0.0 ("AI1 X Set 2")) -> (w434:fxp<+/-,24,9>)
                n228 = Select(t=w421, s=w400, f=w434) -> (s? t:f=w435:fxp<+/-,24,9>)
                "Trap Pos FB Int Signal" <- w435
                n229 = feedback-in #16(w435) -> ()
                n230 = feedback #17(fxp<+/-,16,1> 0.0 ("Trap Pos FB Int-Norm Signal")) -> (w418:fxp<+/-,16,1>)
                n231 = Select(t=w416, s=w400, f=w418) -> (s? t:f=w417:fxp<+/-,16,1>)
                "Trap Pos FB Int-Norm Signal" <- w417
                n232 = feedback-in #17(w417) -> ()
                n233 = case "For position feedback" shown="True" "Force feedback" {
                  tunnel: [i64 0 w482] -> w411
                  tunnel: w416 -> [_ w479]
                  tunnel: w400 -> [_ w478]
                  frame False {
                  }
                  frame True {
                    n234 = feedback #18(i64 0) -> (w481:i64)
                    n235 = case shown="False" w478 {
                      tunnel: [w483 w497] -> w482
                      tunnel: w481 -> [w483 _]
                      tunnel: w479 -> [_ w491]
                      frame False {
                      }
                      frame True {
                        w501 = u32 0
                        n236 = Bundle("P2"="P2", "I2"="I2", "D2"="D2") -> (w487:T8)  [unwired: 1 in]
                        n237 = Bundle("FB2 output high"="FB2 output high", "FB2 output low"="FB2 output low") -> (w484:T9)  [unwired: 1 in]
                        n238 = xnode ("PID")("process variable"=w491, "reset?"="Trap Pos. FB Reset", "setpoint"="Trap Pos. FB SP", "PID gains"=w487, "output range"=w484) -> ("output"=w513:fxp<+/-,16,1>)
                        n239 = Negate(x=w513) -> (-x=w512:fxp<+/-,17,2>)
                        n240 = Select(t=w512, s="Trap Pos FB Negate Action", f=w513) -> (s? t:f=w509:fxp<+/-,17,2>)
                        n241 = Scale By Power Of 2(n=u32 15, x=u32 1) -> (x*2^n=w506:u32)
                        n242 = Multiply(x=w509, y=w506) -> (x*y=w505:fxp<+/-,17,17>)
                        n243 = To Quad Integer(1:w505) -> (0:w517:i64)
                        "Trap Pos FB Action" <- w517
                        n244 = Multiply(x=w517, y="Trap Pos. FB Mult Factor") -> (x*y=w515:i64)
                        n245 = Add(x=w515, y="Trap Pos. FB Offset Factor") -> (x+y=w497:i64)
                        n246 = feedback #19() -> (w498:i64)  [unwired: 1 in]
                        n247 = Add(x=w497, y=w498) -> (x+y=w495:i64)
                        n248 = feedback #20(w501) -> (w503:u32)
                        n249 = Increment(x=w503) -> (x+1=w492:u32)
                        n250 = Greater Or Equal?(x=w492, y="FB Trig Integrate") -> (x >= y?=w493:bool)
                        n251 = Select(t=i64 0, s=w493, f=w495) -> (s? t:f=w499:i64)
                        n252 = feedback-in #19(w499) -> ()
                        n253 = Select(t=w501, s=w493, f=w492) -> (s? t:f=w502:u32)
                        n254 = feedback-in #20(w502) -> ()
                        n255 = And(x=w493, y="FPGA Trap Trig") -> (x .and. y?=w500:bool)
                        n256 = case "Trap FB trigger excitation laser ON" shown="True" w500 {
                          tunnel: w495 -> [_ w521]
                          tunnel: w492 -> [_ w519]
                          frame False {
                          }
                          frame True {
                            n257 = Not(x="TTrig Negate Pos") -> (.not. x?=w528:bool)
                            n258 = Boolean To (0,1)(Boolean="TTrig Negate Pos") -> (0, 1=w526:i16)
                            n259 = Boolean To (0,1)(Boolean=w528) -> (0, 1=w527:i16)
                            n260 = Negate(x=w526) -> (-x=w525:i16)
                            n261 = Add(x=w525, y=w527) -> (x+y=w524:i16)
                            n262 = Multiply(x=w524, y=w521) -> (x*y=w523:i64)
                            "TTrig Sig" <- w523
                            n263 = Multiply(x="FPGA TTrig Thresh", y=w519) -> (x*y=w520:i64)
                            "TTrig Fin Thresh" <- w520
                            n264 = Greater Or Equal?(x=w523, y=w520) -> (x >= y?=w522:bool)
                            n265 = case shown="True" w522 {
                              frame False {
                              }
                              frame True {
                                w531 = TRUE ("Green FB On/Off")
                                w533 = u8 2 ("Operating Mode")
                                n266 = local write "Operating Mode 2"(w533) -> ()
                                n267 = local write "Operating Mode"(w533) -> ()
                                n268 = local write "Green FB On/Off"(w531) -> ()
                                n269 = local write "FPGA Trap Trig"(FALSE ("FPGA Trap Trig")) -> ()
                                "TTrig?" <- w531
                              }
                            }
                          }
                        }
                      }
                    }
                    n270 = feedback-in #18(w482) -> ()
                  }
                }
                n271 = case shown="True" "Dynamic Force FB (Ronen)" {
                  tunnel: w411 -> [w454 w458]
                  tunnel: [w453 w457] -> w409
                  tunnel: w402 -> [_ w456]
                  tunnel: w400 -> [_ w455]
                  frame False {
                    # "(BD1 Frequency 1)"
                    n272 = Add(x="BD 1 Frequency 1", y=w454) -> (x+y=w453:u64)
                  }
                  frame True {
                    n273 = case shown="True" w455 {
                      tunnel: w458 -> [_ w462]
                      tunnel: [w459 w461] -> w457
                      tunnel: w456 -> [w459 w460]
                      frame False {
                      }
                      frame True {
                        n274 = Add(x=w460, y=w462) -> (x+y=w461:u64)
                      }
                    }
                  }
                }
                n275 = Select(t=w443, s="Scan BD", f=w444) -> (s? t:f=w442:u64)
                n276 = Select(t=w444, s="Scan BD", f=w443) -> (s? t:f=w445:u64)
                n277 = Add(x=w442, y="BD 2 Frequency 1") -> (x+y=w447:u64)
                n278 = Compound Arithmetic op=ADD(i64 0 ("f"), w409, w445) -> (w401:u64)
                "BD1 Frequency Out 1" <- w401
              }
              frame 2 {
                # "Trap 2"
                n279 = case shown="True" "FB On/Off Set 2" {
                  tunnel: ["BD 1 Amplitude 2" w664] -> w646
                  tunnel: w647 -> [_ w662]
                  tunnel: w654 -> [_ w667]
                  tunnel: w653 -> [_ w666]
                  tunnel: w650 -> [_ w665]
                  tunnel: w649 -> [_ w663]
                  tunnel: w645 -> [_ w661]
                  tunnel: w644 -> [_ w660]
                  frame False {
                  }
                  frame True {
                    n280 = local read "AI2 Y Sum Set 2"() -> (w669:i16)
                    n281 = case shown="False" w663 {
                      tunnel: "FB Setpoint Set 2" -> [w675 w691]
                      tunnel: w669 -> [w676 w690]
                      tunnel: "FB Reset Set 2" -> [w677 w689]
                      tunnel: w667 -> [w673 w687]
                      tunnel: w666 -> [w674 w686]
                      tunnel: w665 -> [_ w685]
                      tunnel: [w671 w684] -> w664
                      tunnel: w662 -> [_ w683]
                      tunnel: w661 -> [_ w682]
                      tunnel: w660 -> [_ w679]
                      frame False {
                        n282 = call "Slower PID.vi"("process variable"=w676, "reset?"=w677, "setpoint"=w675, "PID gains (x 2^8)"=w673, "output range"=w674) -> ("output"=w672:i16)  [unwired: 10 out]
                        n283 = To Unsigned Word Integer(number=w672) -> (unsigned 16bit integer=w671:u16)
                      }
                      frame True {
                        n284 = call "Slower PID.vi"("process variable"=w690, "reset?"=w689, "setpoint"=w691, "PID gains (x 2^8)"=w687, "output range"=w686) -> ("output"=w688:i16)  [unwired: 10 out]
                        n285 = To Unsigned Word Integer(number=w688) -> (unsigned 16bit integer=w681:u16)
                        n286 = Scale By Power Of 2(n=w682, x=w681) -> (x*2^n=w680:u16)
                        n287 = Add(x=w680, y=w679) -> (x+y=w678:u16)
                        n288 = case shown="False" w685 {
                          tunnel: w683 -> [w693 w697]
                          tunnel: w678 -> [w692 w696]
                          tunnel: [w694 w695] -> w684
                          frame False {
                            n289 = Add(x=w693, y=w692) -> (x+y=w694:u16)
                          }
                          frame True {
                            n290 = Subtract(x=w697, y=w696) -> (x-y=w695:u16)
                          }
                        }
                      }
                    }
                  }
                }
                n291 = Add(x="BD 1 Frequency 2", y=i64 0 ("f")) -> (x+y=w652:u64)
                "BD1 Frequency Out 2" <- w652
              }
              frame 3 {
                # "Fluorescence period"
              }
            }
            n292 = feedback-in #21(w313) -> ()
            n293 = feedback #21(w313) -> (w312:u16)
            n294 = Select(t=w315, s="Interlace ON/OFF", f="Interlace Off Parameters") -> (s? t:f=w352:u8)
            n295 = Subtract(x=w313, y=w312) -> (x-y=w311:u16)
            n296 = Subtract "The error"(x=w311, y=w310) -> (x-y=w288:u16)
            n297 = case shown="1, Default" w352 {
              tunnel: ["DIO count 1 (ticks)" "DIO count 2 (ticks)" "DIO count 3 (ticks)"] -> w309
              frame 1, Default {
              }
              frame 2 {
              }
              frame 3 {
              }
            }
            n298 = Number To Boolean Array(number=w288) -> (Boolean array=w289:bool[])
            n299 = Or Array Elements(Boolean array=w289) -> (logical OR=w287:bool)
            n300 = Boolean To (0,1)(Boolean=w287) -> (0, 1=w294:i16)
            n301 = To Unsigned Byte Integer(number=w294) -> (unsigned 8bit integer=w291:u8)
            n302 = feedback #22(u8 0) -> (w292:u8)
            n303 = Add(x=w291, y=w292) -> (x+y=w290:u8)
            "DIO Late Counter" <- w290
            n304 = feedback-in #22(w290) -> ()
            n305 = Subtract(x=w309, y=w288) -> (x-y=w308:u16)
            n306 = Split Number(x=w349) -> (hi(x)=w348:u32, lo(x)=w347:u32)
            n307 = Split Number(x=w338) -> (hi(x)=w343:u32, lo(x)=w342:u32)
            n308 = Boolean To (0,1)(Boolean="+ phase (DIO)") -> (0, 1=w305:i16)
            n309 = Split Number(x=w348) -> (lo(x)=w346:u16)  [unwired: 1 out]
            n310 = Split Number(x=w347) -> (hi(x)=w345:u16, lo(x)=w344:u16)
            n311 = Split Number(x=w343) -> (lo(x)=w341:u16)  [unwired: 1 out]
            n312 = Split Number(x=w342) -> (hi(x)=w340:u16, lo(x)=w339:u16)
            n313 = Split Number(x=w298) -> (hi(x)=w300:u8, lo(x)=w299:u8)
            n314 = Split Number(x=w295) -> (hi(x)=w297:u8, lo(x)=w296:u8)
            n315 = Split Number(x=w346) -> (hi(x)=w337:u8, lo(x)=w336:u8)
            n316 = Split Number(x=w345) -> (hi(x)=w335:u8, lo(x)=w334:u8)
            n317 = Split Number(x=w341) -> (hi(x)=w330:u8, lo(x)=w329:u8)
            n318 = Split Number(x=w344) -> (hi(x)=w333:u8, lo(x)=w332:u8)
            n319 = Split Number(x=w340) -> (hi(x)=w328:u8, lo(x)=w327:u8)
            n320 = Split Number(x=w339) -> (hi(x)=w326:u8, lo(x)=w325:u8)
            n321 = Multiply(x=w305, y="Phase count adjustment (DIO)") -> (x*y=w301:i16)
            n322 = feedback #23(i16 0) -> (w303:i16)
            n323 = Subtract(x=w303, y=w301) -> (x-y=w302:i16)
            "DIO Relative phase" <- w302
            n324 = feedback-in #23(w302) -> ()
            n325 = Add(x=w308, y=w301) -> (x+y=w307:u16)
            n326 = Build Array "BD 1 A Stack"(w300, w299) -> (w322:u8[])
            n327 = Build Array "BD 2 A Stack"(w297, w296) -> (w321:u8[])
            n328 = Build Array "BD 1 nu Stack"(w337, w336, w335, w334, w333, w332) -> (w331:u8[])
            n329 = Build Array "BD 2 nu Stack"(w330, w329, w328, w327, w326, w325) -> (w324:u8[])
            n330 = case shown="2" w279 {
              tunnel: [w392 w395] -> w320
              tunnel: [u8 10 u8 4] -> w323
              tunnel: "Swap F1 and F2" -> [w393 w395]
              frame 2 {
                # "F2"
                n331 = Not(x=w393) -> (.not. x?=w392:bool)
              }
              frame 1, Default {
                # "low chooses F1"
                # "F1"
              }
            }
            n332 = case "If FPGA is controlling (toggling) RF synth" shown="True" w319 {
              tunnel: w331 -> [_ w368]
              tunnel: w324 -> [_ w367]
              tunnel: w323 -> [_ w366]
              tunnel: w322 -> [_ w365]
              tunnel: w321 -> [_ w364]
              frame False {
              }
              frame True {
                # "Write next amp.\n(wait until beginning of next loop iteration to update)"
                n333 = flat-sequence "Update the next F1 and F2 frequency value (the actual frequency won't change until FSK is switched).\nThen load the next amplitude value into buffer, but don't update it until the next cycle." {
                  tunnel: w367 -> [w370]
                  tunnel: w368 -> [w371]
                  tunnel: [w371] -> w363
                  tunnel: [w370] -> w362
                  tunnel: w366 -> [w372]
                  tunnel: w363 -> [w374]
                  tunnel: w362 -> [w373]
                  tunnel: w365 -> [w385]
                  tunnel: w364 -> [w384]
                  frame #0 {
                    # "To possibly send\nthese writes to very\nend of loop (for x and\ny phase adjust)"
                    n334 = call "Wait8"("Count(Ticks)"="Next trap write delay (ticks)") -> ()  [unwired: 1 out]
                  }
                  frame #1 {
                    n335 = for {
                      tunnel: w374 -> [w380] mode=indexing
                      tunnel: w373 -> [w379] mode=indexing
                      tunnel: w372 -> [w377]
                      i -> [w378]
                      # "Write next freq."
                      n336 = To Unsigned Byte Integer(number=w378) -> (unsigned 8bit integer=w375:u8)
                      n337 = Add(x=w377, y=w375) -> (x+y=w376:u8)
                      n338 = call "write to RF synth bd.vi"("Address Byte"=w376, "BD 2 Byte"=w379, "BD 1 Byte"=w380) -> ()
                    }
                  }
                  frame #2 {
                    w381 = TRUE ("Connector1/DIO15")
                    # "send udclk high\n(BD 1 and 2)"
                    n339 = xnode "FPGA I/O Node"("Connector1/DIO30"=w381, "Connector1/DIO29"=w381) -> ()  [unwired: 2 in, 2 out]
                  }
                  frame #3 {
                    w382 = FALSE ("Connector1/DIO15")
                    n340 = xnode "FPGA I/O Node"("Connector1/DIO30"=w382, "Connector1/DIO29"=w382) -> ()  [unwired: 2 in, 2 out]
                  }
                  frame #4 {
                    n341 = for {
                      tunnel: w385 -> [w391] mode=indexing
                      tunnel: w384 -> [w390] mode=indexing
                      tunnel: u8 33 -> [w388]
                      i -> [w389]
                      n342 = To Unsigned Byte Integer(number=w389) -> (unsigned 8bit integer=w386:u8)
                      n343 = Add(x=w388, y=w386) -> (x+y=w387:u8)
                      n344 = call "write to RF synth bd.vi"("Address Byte"=w387, "BD 2 Byte"=w390, "BD 1 Byte"=w391) -> ()
                    }
                  }
                }
              }
            }
          }
        }
      }
    }
  }
  n345 = while "APD 1 Counter" {
    tunnel: w4 -> [_]
    stop <- FALSE stop-if-true
    n346 = flat-sequence {
      frame #0 {
        n347 = xnode "FPGA I/O Method Node"("FPGA I/O In"=refnum<k21> "Connector0/DIO0" ("APD 1 DO"), "Timeout"=-1) -> ()  [unwired: 2 out]
      }
      frame #1 {
        n348 = local read "APD1 int gate"() -> (w708:bool)
        n349 = case shown="True" w708 {
          frame False {
          }
          frame True {
            n350 = local read "APD1 out state"() -> (w709:bool)
            n351 = case shown="True" w709 {
              frame False {
                n352 = local read "APD 1 Counts 0"() -> (w711:u32)
                n353 = Increment(x=w711) -> (x+1=→"APD 1 Counts 0":u32)
              }
              frame True {
                n354 = local read "APD 1 Counts 1"() -> (w713:u32)
                n355 = Increment(x=w713) -> (x+1=→"APD 1 Counts 1":u32)
              }
            }
          }
        }
      }
    }
  }
  n356 = disable-structure shown="Disabled" {
    disable-tunnel: u16 0 -> [w715 _]
    disable-tunnel: w4 -> [w714 _]
    frame Disabled {
      n357 = while "Green and red fluorescent laser interlacing (Current AO to IA 532 nm AOM ME amp)." {
        shift-right: [w724] -> _
        shift-left: w714 -> [w727]
        shift-right: [w721] -> _
        shift-left: w715 -> [w719]
        shift-right: [w718] -> _
        shift-left: w715 -> [w717]
        stop <- FALSE stop-if-true
        n358 = flat-sequence {
          tunnel: w727 -> [w731]
          tunnel: [w732] -> w726
          tunnel: [w731] -> w725
          tunnel: [w730] -> w720
          tunnel: w719 -> [w730]
          tunnel: w717 -> [w729]
          tunnel: [w729] -> w716
          tunnel: [w736] -> w723
          tunnel: w726 -> [w736]
          tunnel: [w735] -> w722
          tunnel: w725 -> [w735]
          tunnel: w720 -> [w734]
          tunnel: w716 -> [w733]
          tunnel: [w757] -> w724
          tunnel: [w773] -> w721
          tunnel: w723 -> [w784]
          tunnel: w722 -> [w781]
          tunnel: [w741] -> w718
          frame #0 {
            n359 = call "Loop Timer10"("Count(Ticks)"=w731) -> ("Tick Count(Ticks)"=w732:u16)
          }
          frame #1 {
            n360 = xnode "FPGA I/O Node"("Chassis2/Mod1/AO0"=w734, "Chassis2/Mod1/AO1"=w733) -> ()  [unwired: 2 in, 2 out]
          }
          frame #2 {
            # "Design note:\n\nThese two laser controls are in the same loop\nbecause the expansion current AI cannot separately\ntime the outputs fast enough for us.  Apparently\nit is because of communication time between the\nexpansion card and the fpga.\n\nSo the two analog control signals have the same timing\nand profile, but independent amplitudes to independently\ncontrol the intensity and feedback for each laser."
            n361 = feedback #24(TRUE) -> (w737:bool)
            n362 = Not(x=w737) -> (.not. x?=w738:bool)
            n363 = feedback-in #24(w738) -> ()
            n364 = Subtract(x="Green interlace OFF count 2", y="Green int current ON count adj") -> (x-y=w766:u16)
            n365 = feedback-in #25(w784) -> ()
            n366 = feedback #25(w784) -> (w783:u16)
            n367 = Add(x="Green int current ON count adj", y="Green interlace ON count 2") -> (x+y=w767:u16)
            n368 = Subtract(x=w784, y=w783) -> (x-y=w782:u16)
            n369 = Select(t=w767, s=w738, f=w766) -> (s? t:f=w778:u16)
            n370 = Subtract(x=w782, y=w781) -> (x-y=w750:u16)
            n371 = case shown="2" "RI Operating Mode 2" {
              tunnel: [TRUE FALSE w790] -> w739
              tunnel: w737 -> [_ _ w787]
              frame 0, Default {
              }
              frame 1 {
              }
              frame 2 {
                n372 = Not(x=w787) -> (.not. x?=w789:bool)
                n373 = Select(t=w789, s="Invert RI 2", f=w787) -> (s? t:f=w790:bool)
              }
            }
            n374 = Subtract(x=w778, y=w750) -> (x-y=w761:u16)
            n375 = case shown="0, Default" "Operating Mode 2" {
              tunnel: [TRUE FALSE w824] -> w742
              tunnel: w737 -> [_ _ w821]
              frame 0, Default {
              }
              frame 1 {
              }
              frame 2 {
                n376 = Not(x=w821) -> (.not. x?=w823:bool)
                n377 = Select(t=w823, s="Invert GI 2", f=w821) -> (s? t:f=w824:bool)
              }
            }
            n378 = Number To Boolean Array(number=w750) -> (Boolean array=w751:bool[])
            n379 = Boolean To (0,1)(Boolean="+ phase (GI) 2") -> (0, 1=w763:i16)
            n380 = Or Array Elements(Boolean array=w751) -> (logical OR=w749:bool)
            n381 = Boolean To (0,1)(Boolean=w749) -> (0, 1=w756:i16)
            n382 = Multiply(x=w763, y="Phase count adjustment (GI) 2") -> (x*y=w759:i16)
            n383 = To Unsigned Byte Integer(number=w756) -> (unsigned 8bit integer=w752:u8)
            n384 = Add(x=w761, y=w759) -> (x+y=w757:u16)
            n385 = feedback #26(u8 0) -> (w754:u8)
            n386 = Add(x=w752, y=w754) -> (x+y=w753:u8)
            "GI Late Counter 2" <- w753
            n387 = feedback-in #26(w753) -> ()
            n388 = feedback #27(i16 0) -> (w760:i16)
            n389 = Subtract(x=w760, y=w759) -> (x-y=w758:i16)
            "GI Relative phase 2" <- w758
            n390 = feedback-in #27(w758) -> ()
            n391 = And(x=w742, y="Green FB On/Off") -> (x .and. y?=w768:bool)
            n392 = And(x=w739, y="Red FB On/Off") -> (x .and. y?=w748:bool)
            n393 = case shown="False" w768 {
              tunnel: "Current Out" -> [w805 _]
              tunnel: [w805 w814] -> w772
              frame False {
              }
              frame True {
                n394 = local read "Green FB Sum"() -> (w810:i16)
                n395 = Bundle("P3"="P3", "I3"="I3", "D3"="D3") -> (w806:cluster{"P3":i16, "I3":i16, "D3":i16})  [unwired: 1 in]
                n396 = call "Slower PID.vi"("process variable"=w810, "reset?"="Green FB Reset", "setpoint"="Green FB Setpoint", "PID gains (x 2^8)"=w806, "output range"=cluster{"output high":i16, "output low":i16} {"output high"=32767, "output low"=-32768} ("Green FB output range")) -> ("output"=w817:i16)  [unwired: 10 out]
                n397 = To Long Integer(number=w817) -> (32bit integer=w811:i32)
                n398 = Add(x=w811, y=32768) -> (x+y=w813:i32)
                n399 = To Unsigned Word Integer(number=w813) -> (unsigned 16bit integer=w814:u16)
              }
            }
            n400 = case shown="True" w748 {
              tunnel: "RI Current Out" -> [w791 _]
              tunnel: [w791 w800] -> w744
              frame False {
              }
              frame True {
                n401 = local read "Red FB Intensity"() -> (w796:i16)
                n402 = Bundle("P4"="P4", "I4"="I4", "D4"="D4") -> (w792:cluster{"P4":i16, "I4":i16, "D4":i16})  [unwired: 1 in]
                n403 = call "Slower PID.vi"("process variable"=w796, "reset?"="Red FB Reset", "setpoint"="Red FB Setpoint", "PID gains (x 2^8)"=w792, "output range"=cluster{"output high":i16, "output low":i16} {"output high"=32767, "output low"=-32768} ("Green FB output range")) -> ("output"=w803:i16)  [unwired: 10 out]
                n404 = To Long Integer(number=w803) -> (32bit integer=w797:i32)
                n405 = Add(x=w797, y=32768) -> (x+y=w799:i32)
                n406 = To Unsigned Word Integer(number=w799) -> (unsigned 16bit integer=w800:u16)
              }
            }
            n407 = Boolean To (0,1)(Boolean=w742) -> (0, 1=w774:i16)
            n408 = Boolean To (0,1)(Boolean=w739) -> (0, 1=w743:i16)
            n409 = To Unsigned Word Integer(number=w774) -> (unsigned 16bit integer=w771:u16)
            n410 = To Unsigned Word Integer(number=w743) -> (unsigned 16bit integer=w745:u16)
            n411 = Multiply(x=w771, y=w772) -> (x*y=w773:u16)
            n412 = Multiply(x=w745, y=w744) -> (x*y=w741:u16)
          }
        }
      }
    }
    frame Enabled {
    }
  }
  n413 = while "APD 2 Counter" {
    tunnel: w4 -> [_]
    stop <- FALSE stop-if-true
    n414 = flat-sequence {
      frame #0 {
        n415 = xnode "FPGA I/O Method Node"("FPGA I/O In"=refnum<k21> "Connector0/DIO1" ("APD 2 DO"), "Timeout"=-1) -> ()  [unwired: 2 out]
      }
      frame #1 {
        n416 = local read "APD2 int gate"() -> (w828:bool)
        n417 = case shown="True" w828 {
          frame False {
          }
          frame True {
            n418 = local read "APD2 out state"() -> (w829:bool)
            n419 = case shown="False" w829 {
              frame False {
                n420 = local read "APD 2 Counts 0"() -> (w831:u32)
                n421 = Increment(x=w831) -> (x+1=→"APD 2 Counts 0":u32)
              }
              frame True {
                n422 = local read "APD 2 Counts 1"() -> (w833:u32)
                n423 = Increment(x=w833) -> (x+1=→"APD 2 Counts 1":u32)
              }
            }
          }
        }
      }
    }
  }
  n424 = while "532 nm green fluorescent laser interlacing (DO to IA 532 nm AOM ME amp)." {
    shift-right: [w837] -> _
    shift-left: w4 -> [w842]
    shift-right: [w836] -> _
    shift-left: w5 -> [w834]
    stop <- FALSE stop-if-true
    n425 = flat-sequence {
      tunnel: w842 -> [w845]
      tunnel: [w846] -> w840
      tunnel: [w845] -> w838
      tunnel: [w844] -> w835
      tunnel: w834 -> [w844]
      tunnel: [w849] -> w841
      tunnel: w840 -> [w849]
      tunnel: [w848] -> w839
      tunnel: w838 -> [w848]
      tunnel: w835 -> [w847]
      tunnel: [w858] -> w837
      tunnel: w841 -> [w878]
      tunnel: w839 -> [w875]
      tunnel: [w867] -> w836
      frame #0 {
        n426 = call "Loop Timer4"("Count(Ticks)"=w845) -> ("Tick Count(Ticks)"=w846:u16)
      }
      frame #1 {
        n427 = xnode "FPGA I/O Node"("Connector1/DIO34"=w847, "Connector1/DIO38"=w847, "Connector1/DIO39"=w847) -> ()  [unwired: 3 in, 3 out]
      }
      frame #2 {
        n428 = feedback-in #28(w878) -> ()
        n429 = feedback #28(w878) -> (w877:u16)
        n430 = Subtract(x=w878, y=w877) -> (x-y=w876:u16)
        n431 = Subtract(x=w876, y=w875) -> (x-y=w851:u16)
        n432 = Number To Boolean Array(number=w851) -> (Boolean array=w852:bool[])
        n433 = Or Array Elements(Boolean array=w852) -> (logical OR=w850:bool)
        n434 = Boolean To (0,1)(Boolean="+ phase (GI)") -> (0, 1=w863:i16)
        n435 = Multiply(x=w863, y="Phase count adjustment (GI)") -> (x*y=w860:i16)
        n436 = Boolean To (0,1)(Boolean=w850) -> (0, 1=w857:i16)
        n437 = To Unsigned Byte Integer(number=w857) -> (unsigned 8bit integer=w854:u8)
        n438 = feedback #29(i16 0) -> (w861:i16)
        n439 = feedback #30(u8 0) -> (w855:u8)
        n440 = Add(x=w854, y=w855) -> (x+y=w853:u8)
        "GI Late Counter" <- w853
        n441 = feedback-in #30(w853) -> ()
        n442 = Subtract(x=w861, y=w860) -> (x-y=w859:i16)
        "GI Relative phase" <- w859
        n443 = feedback-in #29(w859) -> ()
        n444 = feedback #31(TRUE) -> (w870:bool)
        n445 = case shown="2" "Operating Mode" {
          tunnel: [TRUE FALSE w884] -> w867
          tunnel: w870 -> [_ _ w881]
          frame 0, Default {
          }
          frame 1 {
          }
          frame 2 {
            n446 = Not(x=w881) -> (.not. x?=w883:bool)
            n447 = Select(t=w883, s="Invert GI", f=w881) -> (s? t:f=w884:bool)
          }
        }
        n448 = Not(x=w870) -> (.not. x?=w866:bool)
        n449 = Select(t="Green interlace ON count", s=w866, f="Green interlace OFF count") -> (s? t:f=w872:u16)
        n450 = Subtract(x=w872, y=w851) -> (x-y=w864:u16)
        n451 = Add(x=w864, y=w860) -> (x+y=w858:u16)
        n452 = feedback-in #31(w866) -> ()
      }
    }
  }
  n453 = while "Excitation laser intensity feedback measurement (all lasers)" {
    shift-right: [w885] -> _
    shift-left: w4 -> [w890]
    stop <- FALSE stop-if-true
    n454 = flat-sequence {
      tunnel: w890 -> [w892]
      tunnel: [w893] -> w888
      tunnel: [w892] -> w886
      tunnel: [w899] -> w889
      tunnel: w888 -> [w899]
      tunnel: [w898] -> w887
      tunnel: w886 -> [w898]
      tunnel: [w911] -> w885
      tunnel: w889 -> [w922]
      tunnel: w887 -> [w919]
      frame #0 {
        n455 = call "Loop Timer9"("Count(Ticks)"=w892) -> ("Tick Count(Ticks)"=w893:u16)
      }
      frame #1 {
        # "Design note:\n\nAll lasers need to be measured at the same \ntime because the AI expansion module\ncannot independently time the measurements\nwithin our requirements: their is dead time.\n\nThis probably wouldn't be an issue with the built\nin AI on the fpga board itself."
        n456 = xnode "FPGA I/O Node"("Connector1/DIO35"=TRUE) -> ("Chassis2/Mod2/AI2"=→"Blue Intensity":i16, "Chassis2/Mod2/AI1"=→"Red FB Intensity":i16, "Chassis2/Mod2/AI0"=→"Green FB Sum":i16)  [unwired: 4 in, 4 out]
      }
      frame #2 {
        n457 = feedback-in #32(w922) -> ()
        n458 = feedback #32(w922) -> (w921:u16)
        n459 = Subtract(x=w922, y=w921) -> (x-y=w920:u16)
        n460 = xnode "FPGA I/O Node"("Connector1/DIO35"=FALSE) -> ()  [unwired: 1 in, 1 out]
        n461 = Subtract(x=w920, y=w919) -> (x-y=w901:u16)
        n462 = Subtract(x="Green FB Count", y=w901) -> (x-y=w915:u16)
        n463 = Number To Boolean Array(number=w901) -> (Boolean array=w902:bool[])
        n464 = Or Array Elements(Boolean array=w902) -> (logical OR=w900:bool)
        n465 = Boolean To (0,1)(Boolean="+ phase (Green FB)") -> (0, 1=w913:i16)
        n466 = Boolean To (0,1)(Boolean=w900) -> (0, 1=w907:i16)
        n467 = Multiply(x=w913, y="Phase count adjustment (Green FB)") -> (x*y=w908:i16)
        n468 = Add(x=w915, y=w908) -> (x+y=w911:u16)
        n469 = To Unsigned Byte Integer(number=w907) -> (unsigned 8bit integer=w904:u8)
        n470 = feedback #33(i16 0) -> (w910:i16)
        n471 = Subtract(x=w910, y=w908) -> (x-y=w909:i16)
        "Green FB Relative Phase" <- w909
        n472 = feedback-in #33(w909) -> ()
        n473 = feedback #34(u8 0) -> (w905:u8)
        n474 = Add(x=w904, y=w905) -> (x+y=w903:u8)
        "Green Late Counter" <- w903
        n475 = feedback-in #34(w903) -> ()
      }
    }
  }
  n476 = while "MCL stage control" {
    shift-right: [w935] -> _
    shift-left: w4 -> [w938]
    shift-right: [w928] -> _
    shift-left: w12 -> [w925]
    shift-right: [w927] -> _
    shift-left: w11 -> [w923]
    stop <- FALSE stop-if-true
    n477 = flat-sequence {
      tunnel: w938 -> [w942]
      tunnel: [w943] -> w934
      tunnel: [w942] -> w932
      tunnel: [w941] -> w926
      tunnel: w925 -> [w941]
      tunnel: [w940] -> w924
      tunnel: w923 -> [w940]
      tunnel: w934 -> [w947]
      tunnel: [w947] -> w933
      tunnel: w932 -> [w946]
      tunnel: [w946] -> w931
      tunnel: w926 -> [w945]
      tunnel: w924 -> [w944]
      tunnel: w933 -> [w955]
      tunnel: w931 -> [w954]
      tunnel: [w955] -> w937
      tunnel: [w954] -> w936
      tunnel: [w953] -> w930
      tunnel: [w952] -> w929
      tunnel: [w1027] -> w935
      tunnel: w937 -> [w1034]
      tunnel: w936 -> [w1031]
      tunnel: w930 -> [w1029]
      tunnel: w929 -> [w1028]
      tunnel: [w1029] -> w928
      tunnel: [w1028] -> w927
      frame #0 {
        n478 = call "Loop Timer5"("Count(Ticks)"=w942) -> ("Tick Count(Ticks)"=w943:u32)
      }
      frame #1 {
        n479 = xnode "FPGA I/O Node"("Connector0/AO1"=w945, "Connector0/AO2"=w944) -> ()  [unwired: 2 in, 2 out]
      }
      frame #2 {
        n480 = local read "Scanning MCL"() -> (w967:bool)
        n481 = Or(x=w967, y="Start scan (MCL)") -> (x .or. y?=w962:bool)
        n482 = Not(x="Abort scan (MCL)") -> (.not. x?=w960:bool)
        n483 = And(x=w960, y=w962) -> (x .and. y?=w959:bool)
        n484 = case "Raster scan" shown="True" w959 {
          tunnel: [w968 w1011] -> w964
          tunnel: "Start scan (MCL)" -> [_ w996]
          tunnel: [w968 w972] -> w948
          frame False {
            w968 = i16 0
            n485 = local write "Scanning MCL"(FALSE ("scanning")) -> ()
          }
          frame True {
            w982 = i16 0
            w981 = u64 0
            # "scan incr."
            # "freq. incr. mult."
            # "count steps"
            # "count number of cycles"
            n486 = feedback #35(w981) -> (w1008:u64)
            n487 = Select(t=w981, s=w996, f=w1008) -> (s? t:f=w1010:u64)
            n488 = Increment(x=w1010) -> (x+1=w1007:u64)
            n489 = Greater?(x="Cycles per step (MCL)", y=w1007) -> (0:w991:bool)
            n490 = Select(t=w1007, s=w991, f=w981) -> (s? t:f=w1006:u64)
            n491 = feedback-in #35(w1006) -> ()
            n492 = feedback #36(w981) -> (w1005:u64)
            n493 = Select(t=w981, s=w996, f=w1005) -> (s? t:f=w1000:u64)
            n494 = Increment(x=w1000) -> (x+1=w1004:u64)
            n495 = Add(x="Scan steps (MCL)", y="Scan steps (MCL)") -> (x+y=w1003:u64)
            n496 = Select(t=w1000, s=w991, f=w1004) -> (s? t:f=w986:u64)
            n497 = Greater?(x=w1003, y=w986) -> (0:w985:bool)
            n498 = Select(t=w986, s=w985, f=w981) -> (s? t:f=w1001:u64)
            n499 = feedback-in #36(w1001) -> ()
            n500 = Equal?(x="Scan steps (MCL)", y=w986) -> (x = y?=w990:bool)
            n501 = Greater?(x="Scan steps (MCL)", y=w1000) -> (0:w999:bool)
            n502 = feedback #37(w982) -> (w1002:i16)
            n503 = Select(t=w982, s=w996, f=w1002) -> (s? t:f=w988:i16)
            n504 = Increment(x=w988) -> (x+1=w998:i16)
            n505 = Decrement(x=w988) -> (x-1=w997:i16)
            n506 = Select(t=w998, s=w999, f=w997) -> (s? t:f=w989:i16)
            n507 = Select(t=w988, s=w990, f=w989) -> (s? t:f=w987:i16)
            n508 = Select(t=w988, s=w991, f=w987) -> (s? t:f=w983:i16)
            n509 = Select(t=w983, s=w985, f=w982) -> (s? t:f=w984:i16)
            n510 = feedback-in #37(w984) -> ()
            n511 = feedback #38(w981) -> (w995:u64)
            n512 = Select(t=w981, s=w996, f=w995) -> (s? t:f=w970:u64)
            n513 = Increment(x=w970) -> (x+1=w992:u64)
            n514 = Select(t=w970, s=w985, f=w992) -> (s? t:f=w971:u64)
            n515 = Greater?(x="Number of scans (MCL)", y=w971) -> (0:w978:bool)
            n516 = Multiply(x="Scan freq.  increment (MCL)", y=w988) -> (x*y=w1011:i16)
            n517 = Select(t=TRUE, s="Cont. Scan (MCL)", f=w978) -> (s? t:f=w977:bool)
            "Scanning MCL" <- w977
            n518 = Select(t=w971, s=w977, f=w981) -> (s? t:f=w993:u64)
            n519 = feedback-in #38(w993) -> ()
            n520 = Increment(x=w971) -> (x+1=→"Scan I (MCL)":u64)
            n521 = To Word Integer(number=w970) -> (16bit integer=w973:i16)
            n522 = Multiply(x=w973, y="Scan freq.  increment (MCL)") -> (x*y=w972:i16)
          }
        }
        n523 = Select(t=w948, s="1D or 2D Scan?", f=i16 0) -> (s? t:f=w949:i16)
        n524 = Select(t=w949, s="MCL Scan Axis", f=w964) -> (s? t:f=w963:i16)
        n525 = Select(t=w964, s="MCL Scan Axis", f=w949) -> (s? t:f=w965:i16)
        n526 = Add(x=w963, y="AO2") -> (x+y=w952:i16)
        n527 = Add(x="AO1", y=w965) -> (x+y=w953:i16)
      }
      frame #3 {
        n528 = feedback-in #39(w1034) -> ()
        n529 = feedback #39(w1034) -> (w1033:u32)
        n530 = Boolean To (0,1)(Boolean="+ phase (MCL)") -> (0, 1=w1025:i16)
        n531 = Subtract(x=w1034, y=w1033) -> (x-y=w1032:u32)
        n532 = Multiply(x=w1025, y="Phase count adjustment (MCL)") -> (x*y=w1021:i16)
        n533 = Subtract(x=w1032, y=w1031) -> (x-y=w1013:u32)
        n534 = Subtract(x="MCL count", y=w1013) -> (x-y=w1023:u32)
        n535 = feedback #40(i16 0) -> (w1022:i16)
        n536 = Subtract(x=w1022, y=w1021) -> (x-y=w1020:i16)
        "MCL Relative Phase" <- w1020
        n537 = feedback-in #40(w1020) -> ()
        n538 = Number To Boolean Array(number=w1013) -> (Boolean array=w1014:bool[])
        n539 = Or Array Elements(Boolean array=w1014) -> (logical OR=w1012:bool)
        n540 = Boolean To (0,1)(Boolean=w1012) -> (0, 1=w1019:i16)
        n541 = Add(x=w1023, y=w1021) -> (x+y=w1027:u32)
        n542 = To Unsigned Byte Integer(number=w1019) -> (unsigned 8bit integer=w1016:u8)
        n543 = feedback #41(u8 0) -> (w1017:u8)
        n544 = Add(x=w1016, y=w1017) -> (x+y=w1015:u8)
        "MCL Late Counter" <- w1015
        n545 = feedback-in #41(w1015) -> ()
      }
    }
  }
  n546 = while "Control APD data integration - stream to host" {
    shift-right: [w1039] -> _
    shift-left: w8 -> [w1044]
    stop <- FALSE stop-if-true
    n547 = flat-sequence {
      tunnel: w1044 -> [w1046]
      tunnel: [w1047] -> w1042
      tunnel: [w1046] -> w1040
      tunnel: [w1057] -> w1043
      tunnel: w1042 -> [w1057]
      tunnel: [w1056] -> w1041
      tunnel: w1040 -> [w1056]
      tunnel: [w1055] -> w1038
      tunnel: [w1054] -> w1037
      tunnel: [w1048] -> w1036
      tunnel: [w1099] -> w1039
      tunnel: w1043 -> [w1109]
      tunnel: w1041 -> [w1106]
      tunnel: w1038 -> [w1092]
      tunnel: w1037 -> [w1091]
      tunnel: w1036 -> [w1079]
      frame #0 {
        n548 = call "Loop Timer6"("Count(Ticks)"=w1046) -> ("Tick Count(Ticks)"=w1047:u32)
      }
      frame #1 {
        n549 = flat-sequence {
          tunnel: [w1059] -> w1053
          tunnel: w1053 -> [w1062]
          tunnel: [w1066] -> w1052
          tunnel: [w1065] -> w1051
          tunnel: [w1062] -> w1050
          tunnel: [w1061] -> w1049
          tunnel: [w1073] -> w1054
          tunnel: [w1074] -> w1055
          tunnel: w1052 -> [w1074]
          tunnel: w1051 -> [w1073]
          tunnel: w1050 -> [w1072]
          tunnel: w1049 -> [w1071]
          tunnel: [w1071] -> w1048
          frame #0 {
            # "use separate variable so each APD won't\nhave to wait to read"
            n550 = feedback #42(FALSE) -> (w1058:bool)
            "APD1 out state" <- w1058
            "APD2 out state" <- w1058
            "APD3 out state" <- w1058
            n551 = Not(x=w1058) -> (.not. x?=w1059:bool)
            n552 = feedback-in #42(w1059) -> ()
          }
          frame #1 {
            n553 = local read "APD 3 Counts 1"() -> (w1064:u32)
            n554 = local read "APD 3 Counts 0"() -> (w1063:u32)
            n555 = local read "APD 1 Counts 1"() -> (w1070:u32)
            n556 = local read "APD 1 Counts 0"() -> (w1069:u32)
            n557 = local read "APD 2 Counts 1"() -> (w1068:u32)
            n558 = local read "APD 2 Counts 0"() -> (w1067:u32)
            n559 = Select(t=w1064, s=w1062, f=w1063) -> (s? t:f=w1061:u32)
            n560 = Select(t=w1070, s=w1062, f=w1069) -> (s? t:f=w1066:u32)
            n561 = Select(t=w1068, s=w1062, f=w1067) -> (s? t:f=w1065:u32)
          }
          frame #2 {
            n562 = case shown="False" w1072 {
              frame False {
                w1075 = u32 0 ("APD 1 Counts 0")
                n563 = local write "APD 1 Counts 0"(w1075) -> ()
                n564 = local write "APD 2 Counts 0"(w1075) -> ()
                n565 = local write "APD 3 Counts 0"(w1075) -> ()
              }
              frame True {
                w1076 = u32 0 ("APD 1 Counts 1")
                n566 = local write "APD 1 Counts 1"(w1076) -> ()
                n567 = local write "APD 2 Counts 1"(w1076) -> ()
                n568 = local write "APD 3 Counts 1"(w1076) -> ()
              }
            }
          }
        }
      }
      frame #2 {
        n569 = feedback-in #43(w1109) -> ()
        n570 = feedback #43(w1109) -> (w1108:u32)
        n571 = Subtract(x=w1109, y=w1108) -> (x-y=w1107:u32)
        n572 = Subtract(x=w1107, y=w1106) -> (x-y=w1084:u32)
        n573 = case shown="True" "APD to FIFO" {
          tunnel: w1092 -> [_ w1114]
          tunnel: w1091 -> [_ w1112]
          tunnel: w1079 -> [_ w1110]
          frame False {
          }
          frame True {
            n574 = flat-sequence {
              tunnel: 0 ("Timeout") -> [w1116]
              tunnel: w1114 -> [w1117]
              tunnel: [w1116] -> w1113
              tunnel: w1113 -> [w1118]
              tunnel: w1112 -> [w1119]
              tunnel: [w1118] -> w1111
              tunnel: w1111 -> [w1121]
              tunnel: w1110 -> [w1120]
              frame #0 {
                n575 = xnode ("FIFO Write")("Element"=w1117, "Timeout"=w1116) -> ()  [unwired: 1 in, 2 out]
              }
              frame #1 {
                n576 = xnode ("FIFO Write")("Element"=w1119, "Timeout"=w1118) -> ()  [unwired: 1 in, 2 out]
              }
              frame #2 {
                n577 = xnode ("FIFO Write")("Element"=w1120, "Timeout"=w1121) -> ()  [unwired: 1 in, 2 out]
              }
            }
          }
        }
        n578 = Subtract(x="APD Acq Rate Count", y=w1084) -> (x-y=w1100:u32)
        n579 = Number To Boolean Array(number=w1084) -> (Boolean array=w1085:bool[])
        n580 = Or Array Elements(Boolean array=w1085) -> (logical OR=w1083:bool)
        n581 = Boolean To (0,1)(Boolean=w1083) -> (0, 1=w1090:i16)
        n582 = To Unsigned Byte Integer(number=w1090) -> (unsigned 8bit integer=w1087:u8)
        n583 = feedback #44(u8 0) -> (w1088:u8)
        n584 = Add(x=w1087, y=w1088) -> (x+y=w1086:u8)
        "APD Acq Late Counter" <- w1086
        n585 = feedback-in #44(w1086) -> ()
        n586 = Boolean To (0,1)(Boolean="+ phase (APD Acq)") -> (0, 1=w1096:i16)
        n587 = Multiply(x=w1096, y="Phase Count Adjustment (APD Acq)") -> (x*y=w1093:i16)
        n588 = Add(x=w1100, y=w1093) -> (x+y=w1099:u32)
        n589 = feedback #45(i16 0) -> (w1098:i16)
        n590 = Subtract(x=w1098, y=w1093) -> (x-y=w1095:i16)
        "APD Acq Relative Phase" <- w1095
        n591 = feedback-in #45(w1095) -> ()
        n592 = To Word Integer(number=w1092) -> (16bit integer=w1101:i16)
        n593 = To Word Integer(number=w1079) -> (16bit integer=w1080:i16)
        n594 = To Word Integer(number=w1091) -> (16bit integer=w1102:i16)
        n595 = Multiply(x="APD AO scale factor", y=w1102) -> (x*y=w1081:i16)
        n596 = Multiply(x="APD AO scale factor", y=w1080) -> (x*y=w1077:i16)
        n597 = Multiply(x="APD AO scale factor", y=w1101) -> (x*y=w1082:i16)
        n598 = xnode "FPGA I/O Node"("Connector0/AO6"=w1082, "Connector0/AO7"=w1081, "Connector0/AO5"=w1077) -> ()  [unwired: 3 in, 3 out]
      }
    }
  }
  n599 = while "DAQ AI set 1" {
    shift-right: [w1122] -> _
    shift-left: w4 -> [w1127]
    stop <- FALSE stop-if-true
    n600 = flat-sequence {
      tunnel: w1127 -> [w1137]
      tunnel: [w1138] -> w1125
      tunnel: [w1137] -> w1124
      tunnel: [w1148] -> w1135
      tunnel: [w1147] -> w1134
      tunnel: [w1146] -> w1133
      tunnel: [w1145] -> w1132
      tunnel: [w1144] -> w1131
      tunnel: [w1143] -> w1130
      tunnel: [w1142] -> w1129
      tunnel: [w1141] -> w1128
      tunnel: [w1140] -> w1126
      tunnel: w1125 -> [w1140]
      tunnel: w1124 -> [w1139]
      tunnel: [w1139] -> w1123
      tunnel: [w1178] -> w1122
      tunnel: w1135 -> [w1204]
      tunnel: w1134 -> [w1170]
      tunnel: w1133 -> [w1171]
      tunnel: w1132 -> [w1150]
      tunnel: w1131 -> [w1194]
      tunnel: w1130 -> [w1193]
      tunnel: w1129 -> [w1192]
      tunnel: w1128 -> [w1191]
      tunnel: w1126 -> [w1188]
      tunnel: w1123 -> [w1185]
      frame #0 {
        n601 = call "Loop Timer3"("Count(Ticks)"=w1137) -> ("Tick Count(Ticks)"=w1138:u16)
      }
      frame #1 {
        n602 = xnode "FPGA I/O Node"("Connector1/DIO31"=TRUE ("Connector1/DIO33")) -> ("Connector0/AI0"=w1148:i16, "Connector0/AI1"=w1147:i16, "Connector0/AI2"=w1146:i16, "Connector0/AI3"=w1145:i16, "Connector0/AI4"=w1144:i16, "Connector0/AI5"=w1143:i16, "Connector0/AI6"=w1142:i16, "Connector0/AI7"=w1141:i16)  [unwired: 9 in, 9 out]
      }
      frame #2 {
        w1174 = FALSE ("AI to FIFO")
        # "Adjust phase after data acquired if button pressed"
        n603 = feedback #46(i16 1) -> (w1197:i16)
        n604 = Increment(x=w1197) -> (x+1=w1203:i16)
        n605 = Scale By Power Of 2(n="AI1 X Scale", x=w1170) -> (x*2^n=w1168:i16)
        n606 = Greater?(x=w1203, y="N of AI1 Int Acq Sets") -> (0:w1200:bool)
        n607 = Select(t=i16 1, s=w1200, f=w1203) -> (s? t:f=w1202:i16)
        n608 = feedback-in #46(w1202) -> ()
        n609 = Divide(x=w1168, y=w1150) -> (x/y=w1167:fxp<+/-,16,1>)
        n610 = feedback #47(w1174) -> (w1172:bool)
        n611 = feedback #48(w1174) -> (w1190:bool)
        n612 = case shown="2" w1197 {
          tunnel: w1171 -> [w1227 w1234 _]
          tunnel: ["Set 1" "Set 2" "Set 3"] -> w1195
          tunnel: ["AI to FIFO" w1236 w1241] -> w1189
          tunnel: w1190 -> [_ w1236 w1241]
          tunnel: ["Trap Pos to FIFO" w1235 w1240] -> w1173
          tunnel: w1172 -> [_ w1235 w1240]
          tunnel: w1167 -> [w1226 w1233 _]
          tunnel: [w1225 w1231 FALSE] -> w1154
          tunnel: [w1224 w1232 u64 0 ("BD1 Frequency Out 2")] -> w1153
          frame 1, Default {
            n613 = local read "BD1 Frequency Out 1"() -> (w1224:u64)
            n614 = Compound Arithmetic op=AND("Trap Pos to FIFO", "Set 1", "AI to FIFO") -> (w1225:bool)
            "AI2 Y Sum Set 1" <- w1227
            "AI1 X Set 1" <- w1226
          }
          frame 2 {
            n615 = local read "BD1 Frequency Out 2"() -> (w1232:u64)
            n616 = Compound Arithmetic op=AND(w1235, "Set 2", w1236) -> (w1231:bool)
            "AI2 Y Sum Set 2" <- w1234
            "AI1 X Set 2" <- w1233
          }
          frame 3 {
          }
        }
        n617 = And(x=w1195, y=w1189) -> (x .and. y?=w1196:bool)
        n618 = case shown="True" w1196 {
          tunnel: w1204 -> [_ w1255]
          tunnel: w1170 -> [_ w1254]
          tunnel: w1171 -> [_ w1253]
          tunnel: w1150 -> [_ w1252]
          tunnel: w1194 -> [_ w1251]
          tunnel: w1193 -> [_ w1250]
          tunnel: w1192 -> [_ w1249]
          tunnel: w1191 -> [_ w1248]
          tunnel: 0 ("DMA buffer timeout") -> [_ w1257]
          frame False {
          }
          frame True {
            n619 = Build Array(w1255, w1254, w1253, w1252, w1251, w1250, w1249, w1248) -> (w1256:i16[])
            n620 = for {
              tunnel: w1256 -> [w1259] mode=indexing
              tunnel: w1257 -> [w1260]
              tunnel: [w1258] -> w1246 mode=indexing
              n621 = xnode ("FIFO Write")("Element"=w1259, "Timeout"=w1260) -> ("Timed Out?"=w1258:bool)  [unwired: 1 in, 1 out]
            }
            n622 = Or Array Elements(Boolean array=w1246) -> (logical OR=w1243:bool)
            n623 = Boolean To (0,1)(Boolean=w1243) -> (0, 1=w1245:i16)
            n624 = feedback #49(u16 0) -> (w1244:u16)
            n625 = Add(x=w1245, y=w1244) -> (x+y=w1242:u16)
            "Trap AI FIFO Timeout" <- w1242
            n626 = feedback-in #49(w1242) -> ()
          }
        }
        n627 = feedback-in #47(w1173) -> ()
        n628 = feedback-in #48(w1189) -> ()
        n629 = case shown="True" w1154 {
          tunnel: w1153 -> [_ w1210]
          tunnel: [u8 0 w1207] -> w1152
          frame False {
          }
          frame True {
            n630 = Split Number(x=w1210) -> (hi(x)=w1211:u32, lo(x)=w1212:u32)
            n631 = Split Number(x=w1211) -> (lo(x)=w1213:u16)  [unwired: 1 out]
            n632 = Split Number(x=w1212) -> (hi(x)=w1214:u16, lo(x)=w1215:u16)
            n633 = Build Array "BD 1 nu Stack"(w1213, w1214, w1215) -> (w1209:u16[])
            n634 = for {
              tunnel: w1209 -> [w1222] mode=indexing
              shift-right: [w1218] -> w1207
              shift-left: u8 0 -> [w1219]
              n635 = xnode ("FIFO Method Node")("Element"=w1222, "Timeout"="Trap FIFO Set Timeout") -> ("Timed Out?"=w1221:bool)  [unwired: 1 in, 1 out]
              n636 = Boolean To (0,1)(Boolean=w1221) -> (0, 1=w1220:i16)
              n637 = To Unsigned Byte Integer(number=w1220) -> (unsigned 8bit integer=w1217:u8)
              n638 = Add(x=w1217, y=w1219) -> (x+y=w1218:u8)
            }
          }
        }
        n639 = To Unsigned Word Integer(number=w1152) -> (unsigned 16bit integer=w1151:u16)
        n640 = feedback #50(u16 0) -> (w1165:u16)
        n641 = Add(x=w1151, y=w1165) -> (x+y=w1164:u16)
        "Trap Pos FIFO Timeout" <- w1164
        n642 = feedback-in #50(w1164) -> ()
        n643 = feedback-in #51(w1188) -> ()
        n644 = feedback #51(w1188) -> (w1187:u16)
        n645 = Subtract(x=w1188, y=w1187) -> (x-y=w1186:u16)
        n646 = xnode "FPGA I/O Node"("Connector1/DIO31"=FALSE ("Connector1/DIO34")) -> ()  [unwired: 1 in, 1 out]
        n647 = Subtract(x=w1186, y=w1185) -> (x-y=w1156:u16)
        n648 = Boolean To (0,1)(Boolean="+ phase") -> (0, 1=w1181:i16)
        n649 = Multiply(x=w1181, y="Phase count adjustment") -> (x*y=w1175:i16)
        n650 = Subtract(x="ai count", y=w1156) -> (x-y=w1179:u16)
        n651 = Number To Boolean Array(number=w1156) -> (Boolean array=w1157:bool[])
        n652 = feedback #52(i16 0) -> (w1177:i16)
        n653 = Add(x=w1179, y=w1175) -> (x+y=w1178:u16)
        n654 = Subtract(x=w1177, y=w1175) -> (x-y=w1176:i16)
        "Relative phase" <- w1176
        n655 = feedback-in #52(w1176) -> ()
        n656 = Or Array Elements(Boolean array=w1157) -> (logical OR=w1155:bool)
        n657 = Boolean To (0,1)(Boolean=w1155) -> (0, 1=w1162:i16)
        n658 = To Unsigned Byte Integer(number=w1162) -> (unsigned 8bit integer=w1159:u8)
        n659 = feedback #53(u8 0) -> (w1160:u8)
        n660 = Add(x=w1159, y=w1160) -> (x+y=w1158:u8)
        "AI Late Counter" <- w1158
        n661 = feedback-in #53(w1158) -> ()
      }
    }
  }
  n662 = node-c288(w9) -> ()
  n663 = while "APD 3 Counter" {
    tunnel: w4 -> [_]
    stop <- FALSE stop-if-true
    n664 = flat-sequence {
      frame #0 {
        n665 = xnode "FPGA I/O Method Node"("FPGA I/O In"=refnum<k21> "Connector0/DIO2" ("APD 2 DO"), "Timeout"=-1) -> ()  [unwired: 2 out]
      }
      frame #1 {
        n666 = local read "APD3 int gate"() -> (w1264:bool)
        n667 = case shown="True" w1264 {
          frame False {
          }
          frame True {
            n668 = local read "APD3 out state"() -> (w1265:bool)
            n669 = case shown="True" w1265 {
              frame False {
                n670 = local read "APD 3 Counts 0"() -> (w1267:u32)
                n671 = Increment(x=w1267) -> (x+1=→"APD 3 Counts 0":u32)
              }
              frame True {
                n672 = local read "APD 3 Counts 1"() -> (w1269:u32)
                n673 = Increment(x=w1269) -> (x+1=→"APD 3 Counts 1":u32)
              }
            }
          }
        }
      }
    }
  }
  n674 = while "APD 3 Gating" {
    shift-right: [w1273] -> _
    shift-left: w4 -> [w1278]
    shift-right: [w1272] -> _
    shift-left: w7 -> [w1270]
    stop <- FALSE stop-if-true
    n675 = flat-sequence {
      tunnel: w1278 -> [w1281]
      tunnel: [w1282] -> w1276
      tunnel: [w1281] -> w1274
      tunnel: [w1280] -> w1271
      tunnel: w1270 -> [w1280]
      tunnel: [w1285] -> w1277
      tunnel: w1276 -> [w1285]
      tunnel: [w1284] -> w1275
      tunnel: w1274 -> [w1284]
      tunnel: w1271 -> [w1283]
      tunnel: [w1306] -> w1273
      tunnel: w1277 -> [w1317]
      tunnel: w1275 -> [w1314]
      tunnel: [w1286] -> w1272
      frame #0 {
        n676 = call "Loop Timer15"("Count(Ticks)"=w1281) -> ("Tick Count(Ticks)"=w1282:u16)
      }
      frame #1 {
        # "Signal maybe then sent through \na transistor before APD"
        n677 = xnode "FPGA I/O Node"("Connector0/DIO12"=w1283, "Connector0/DIO13"=w1283, "Connector0/DIO14"=w1283, "Connector0/DIO15"=w1283) -> ()  [unwired: 4 in, 4 out]
        "APD3 int gate" <- w1283
      }
      frame #2 {
        n678 = local read "APD Gate OFF Count"() -> (w1291:u16)
        n679 = local read "APD Gate ON Count"() -> (w1292:u16)
        n680 = feedback #54(TRUE) -> (w1311:bool)
        n681 = feedback-in #55(w1317) -> ()
        n682 = feedback #55(w1317) -> (w1316:u16)
        n683 = Not(x=w1311) -> (.not. x?=w1309:bool)
        n684 = feedback-in #54(w1309) -> ()
        n685 = Subtract(x=w1317, y=w1316) -> (x-y=w1315:u16)
        n686 = Select(t=w1292, s=w1309, f=w1291) -> (s? t:f=w1313:u16)
        n687 = Subtract(x=w1315, y=w1314) -> (x-y=w1294:u16)
        n688 = Subtract(x=w1313, y=w1294) -> (x-y=w1305:u16)
        n689 = Number To Boolean Array(number=w1294) -> (Boolean array=w1295:bool[])
        n690 = Or Array Elements(Boolean array=w1295) -> (logical OR=w1293:bool)
        n691 = Boolean To (0,1)(Boolean=w1293) -> (0, 1=w1300:i16)
        n692 = Boolean To (0,1)(Boolean="+ phase (APD 3 Gate)") -> (0, 1=w1303:i16)
        n693 = To Unsigned Byte Integer(number=w1300) -> (unsigned 8bit integer=w1297:u8)
        n694 = Multiply(x=w1303, y="Phase count adjustment (APD 3 Gate)") -> (x*y=w1301:i16)
        n695 = feedback #56(u8 0) -> (w1298:u8)
        n696 = Add(x=w1297, y=w1298) -> (x+y=w1296:u8)
        "APD 3 Gate Late Counter" <- w1296
        n697 = feedback-in #56(w1296) -> ()
        n698 = Add(x=w1305, y=w1301) -> (x+y=w1306:u16)
        n699 = feedback #57(i16 0) -> (w1308:i16)
        n700 = Subtract(x=w1308, y=w1301) -> (x-y=w1307:i16)
        "APD 3 Gate Relative Phase" <- w1307
        n701 = feedback-in #57(w1307) -> ()
        n702 = local read "APD Gate Operating Mode"() -> (w1290:u8)
        n703 = case shown="2" w1290 {
          tunnel: [TRUE FALSE w1320] -> w1287
          tunnel: w1311 -> [_ _ w1320]
          frame 0, Default {
          }
          frame 1 {
          }
          frame 2 {
          }
        }
        n704 = local read "Invert APD Gate"() -> (w1289:bool)
        n705 = Not(x=w1287) -> (.not. x?=w1288:bool)
        n706 = Select(t=w1288, s=w1289, f=w1287) -> (s? t:f=w1286:bool)
      }
    }
  }
  n707 = disable-structure shown="Disabled" {
    disable-tunnel: w5 -> [w1322 _]
    disable-tunnel: w4 -> [w1321 _]
    frame Disabled {
      n708 = while "633 nm red  fluorescent laser interlacing (DO to IA 633 nm AOM ME amp)." {
        shift-right: [w1326] -> _
        shift-left: w1321 -> [w1331]
        shift-right: [w1325] -> _
        shift-left: w1322 -> [w1323]
        stop <- FALSE stop-if-true
        n709 = flat-sequence {
          tunnel: w1331 -> [w1334]
          tunnel: [w1335] -> w1329
          tunnel: [w1334] -> w1327
          tunnel: [w1333] -> w1324
          tunnel: w1323 -> [w1333]
          tunnel: [w1338] -> w1330
          tunnel: w1329 -> [w1338]
          tunnel: [w1337] -> w1328
          tunnel: w1327 -> [w1337]
          tunnel: w1324 -> [w1336]
          tunnel: [w1347] -> w1326
          tunnel: w1330 -> [w1367]
          tunnel: w1328 -> [w1364]
          tunnel: [w1356] -> w1325
          frame #0 {
            n710 = call "Loop Timer11"("Count(Ticks)"=w1334) -> ("Tick Count(Ticks)"=w1335:u16)
          }
          frame #1 {
            # "Then to PRL 440 amp"
            n711 = xnode "FPGA I/O Node"("Connector1/DIO32"=w1336) -> ()  [unwired: 1 in, 1 out]
          }
          frame #2 {
            n712 = feedback-in #58(w1367) -> ()
            n713 = feedback #58(w1367) -> (w1366:u16)
            n714 = Subtract(x=w1367, y=w1366) -> (x-y=w1365:u16)
            n715 = Subtract(x=w1365, y=w1364) -> (x-y=w1340:u16)
            n716 = Number To Boolean Array(number=w1340) -> (Boolean array=w1341:bool[])
            n717 = Or Array Elements(Boolean array=w1341) -> (logical OR=w1339:bool)
            n718 = Boolean To (0,1)(Boolean="+ phase (RI)") -> (0, 1=w1352:i16)
            n719 = Multiply(x=w1352, y="Phase count adjustment (RI)") -> (x*y=w1349:i16)
            n720 = Boolean To (0,1)(Boolean=w1339) -> (0, 1=w1346:i16)
            n721 = To Unsigned Byte Integer(number=w1346) -> (unsigned 8bit integer=w1343:u8)
            n722 = feedback #59(i16 0) -> (w1350:i16)
            n723 = feedback #60(u8 0) -> (w1344:u8)
            n724 = Add(x=w1343, y=w1344) -> (x+y=w1342:u8)
            "RI Late Counter" <- w1342
            n725 = feedback-in #60(w1342) -> ()
            n726 = Subtract(x=w1350, y=w1349) -> (x-y=w1348:i16)
            "RI Relative phase" <- w1348
            n727 = feedback-in #59(w1348) -> ()
            n728 = feedback #61(TRUE) -> (w1359:bool)
            n729 = case shown="2" "Red Laser Operating Mode" {
              tunnel: [TRUE FALSE w1373] -> w1356
              tunnel: w1359 -> [_ _ w1370]
              frame 0, Default {
              }
              frame 1 {
              }
              frame 2 {
                n730 = Not(x=w1370) -> (.not. x?=w1372:bool)
                n731 = Select(t=w1372, s="Invert RI", f=w1370) -> (s? t:f=w1373:bool)
              }
            }
            n732 = Not(x=w1359) -> (.not. x?=w1355:bool)
            n733 = Select(t="Red interlace ON count", s=w1355, f="Red interlace OFF count") -> (s? t:f=w1361:u16)
            n734 = Subtract(x=w1361, y=w1340) -> (x-y=w1353:u16)
            n735 = Add(x=w1353, y=w1349) -> (x+y=w1347:u16)
            n736 = feedback-in #61(w1355) -> ()
          }
        }
      }
    }
    frame Enabled {
    }
  }
  n737 = disable-structure shown="Disabled" {
    disable-tunnel: w4 -> [w1374 _]
    frame Disabled {
      n738 = while "Blue fluorescent laser interlacing (AO control direct to laser)." {
        shift-right: [w1381] -> _
        shift-left: w1374 -> [w1384]
        shift-right: [w1378] -> _
        shift-left: i16 0 -> [w1376]
        stop <- FALSE stop-if-true
        n739 = flat-sequence {
          tunnel: w1384 -> [w1387]
          tunnel: [w1388] -> w1383
          tunnel: [w1387] -> w1382
          tunnel: [w1386] -> w1377
          tunnel: w1376 -> [w1386]
          tunnel: [w1391] -> w1380
          tunnel: w1383 -> [w1391]
          tunnel: [w1390] -> w1379
          tunnel: w1382 -> [w1390]
          tunnel: w1377 -> [w1389]
          tunnel: [w1401] -> w1381
          tunnel: [w1417] -> w1378
          tunnel: w1380 -> [w1429]
          tunnel: w1379 -> [w1426]
          frame #0 {
            n740 = call "Loop Timer13"("Count(Ticks)"=w1387) -> ("Tick Count(Ticks)"=w1388:u16)
          }
          frame #1 {
            n741 = xnode "FPGA I/O Node"("Connector0/AO3"=w1389) -> ()  [unwired: 1 in, 1 out]
          }
          frame #2 {
            n742 = Subtract(x="Blue OFF count (AO)", y="Blue current ON count adj (AO)") -> (x-y=w1410:u16)
            n743 = feedback-in #62(w1429) -> ()
            n744 = feedback #62(w1429) -> (w1428:u16)
            n745 = Add(x="Blue current ON count adj (AO)", y="Blue ON count (AO)") -> (x+y=w1411:u16)
            n746 = Subtract(x=w1429, y=w1428) -> (x-y=w1427:u16)
            n747 = Subtract(x=w1427, y=w1426) -> (x-y=w1394:u16)
            n748 = Number To Boolean Array(number=w1394) -> (Boolean array=w1395:bool[])
            n749 = Boolean To (0,1)(Boolean="+ phase (BI AO)") -> (0, 1=w1407:i16)
            n750 = Or Array Elements(Boolean array=w1395) -> (logical OR=w1393:bool)
            n751 = Boolean To (0,1)(Boolean=w1393) -> (0, 1=w1400:i16)
            n752 = Multiply(x=w1407, y="Phase count adjustment (BI AO)") -> (x*y=w1403:i16)
            n753 = To Unsigned Byte Integer(number=w1400) -> (unsigned 8bit integer=w1396:u8)
            n754 = feedback #63(u8 0) -> (w1398:u8)
            n755 = Add(x=w1396, y=w1398) -> (x+y=w1397:u8)
            "BI Late Counter (AO)" <- w1397
            n756 = feedback-in #63(w1397) -> ()
            n757 = feedback #64(i16 0) -> (w1404:i16)
            n758 = Subtract(x=w1404, y=w1403) -> (x-y=w1402:i16)
            "BI Relative phase (AO)" <- w1402
            n759 = feedback-in #64(w1402) -> ()
            n760 = feedback #65(TRUE) -> (w1421:bool)
            n761 = case shown="2" "BI Operating Mode (AO)" {
              tunnel: [TRUE FALSE w1445] -> w1412
              tunnel: w1421 -> [_ _ w1442]
              frame 0, Default {
              }
              frame 1 {
              }
              frame 2 {
                n762 = Not(x=w1442) -> (.not. x?=w1444:bool)
                n763 = Select(t=w1444, s="Invert BI (AO)", f=w1442) -> (s? t:f=w1445:bool)
              }
            }
            n764 = And(x=w1412, y="Blue FB On/Off") -> (x .and. y?=w1413:bool)
            n765 = case shown="True" w1413 {
              tunnel: "BI Current Out" -> [w1430 _]
              tunnel: [w1430 w1432] -> w1416
              frame False {
              }
              frame True {
                n766 = local read "Blue Intensity"() -> (w1431:i16)
                n767 = Bundle("P5"="P5", "I5"="I5", "D5"="D5") -> (w1433:cluster{"P5":i16, "I5":i16, "D5":i16})  [unwired: 1 in]
                n768 = call "Slower PID.vi"("process variable"=w1431, "reset?"="Blue FB Reset", "setpoint"="Blue FB Setpoint", "PID gains (x 2^8)"=w1433, "output range"=cluster{"output high":i16, "output low":i16} {"output high"=32767, "output low"=0} ("Green FB output range")) -> ("output"=w1432:i16)  [unwired: 10 out]
              }
            }
            n769 = Not(x=w1421) -> (.not. x?=w1418:bool)
            n770 = Select(t=w1411, s=w1418, f=w1410) -> (s? t:f=w1423:u16)
            n771 = Subtract(x=w1423, y=w1394) -> (x-y=w1405:u16)
            n772 = Add(x=w1405, y=w1403) -> (x+y=w1401:u16)
            n773 = feedback-in #65(w1418) -> ()
            n774 = Boolean To (0,1)(Boolean=w1412) -> (0, 1=w1392:i16)
            n775 = Multiply(x=w1392, y=w1416) -> (x*y=w1417:i16)
          }
        }
      }
    }
    frame Enabled {
    }
  }
  n776 = disable-structure shown="Disabled" {
    disable-tunnel: w5 -> [w1447 _]
    disable-tunnel: w4 -> [w1446 _]
    frame Disabled {
      n777 = while "473 nm blue  fluorescent laser interlacing (DO to blue laser digital control input)." {
        shift-right: [w1451] -> _
        shift-left: w1446 -> [w1456]
        shift-right: [w1450] -> _
        shift-left: w1447 -> [w1448]
        stop <- FALSE stop-if-true
        n778 = flat-sequence {
          tunnel: w1456 -> [w1459]
          tunnel: [w1460] -> w1454
          tunnel: [w1459] -> w1452
          tunnel: [w1458] -> w1449
          tunnel: w1448 -> [w1458]
          tunnel: [w1463] -> w1455
          tunnel: w1454 -> [w1463]
          tunnel: [w1462] -> w1453
          tunnel: w1452 -> [w1462]
          tunnel: w1449 -> [w1461]
          tunnel: [w1472] -> w1451
          tunnel: w1455 -> [w1492]
          tunnel: w1453 -> [w1489]
          tunnel: [w1481] -> w1450
          frame #0 {
            n779 = call "Loop Timer14"("Count(Ticks)"=w1459) -> ("Tick Count(Ticks)"=w1460:u16)
          }
          frame #1 {
            n780 = xnode "FPGA I/O Node"("Connector1/DIO28"=w1461) -> ()  [unwired: 1 in, 1 out]
          }
          frame #2 {
            n781 = feedback-in #66(w1492) -> ()
            n782 = feedback #66(w1492) -> (w1491:u16)
            n783 = Subtract(x=w1492, y=w1491) -> (x-y=w1490:u16)
            n784 = Subtract(x=w1490, y=w1489) -> (x-y=w1465:u16)
            n785 = Number To Boolean Array(number=w1465) -> (Boolean array=w1466:bool[])
            n786 = Or Array Elements(Boolean array=w1466) -> (logical OR=w1464:bool)
            n787 = Boolean To (0,1)(Boolean="+ phase (BI D)") -> (0, 1=w1477:i16)
            n788 = Multiply(x=w1477, y="Phase count adjustment (BI D)") -> (x*y=w1474:i16)
            n789 = Boolean To (0,1)(Boolean=w1464) -> (0, 1=w1471:i16)
            n790 = To Unsigned Byte Integer(number=w1471) -> (unsigned 8bit integer=w1468:u8)
            n791 = feedback #67(i16 0) -> (w1475:i16)
            n792 = feedback #68(u8 0) -> (w1469:u8)
            n793 = Add(x=w1468, y=w1469) -> (x+y=w1467:u8)
            "Blue Late Counter (D)" <- w1467
            n794 = feedback-in #68(w1467) -> ()
            n795 = Subtract(x=w1475, y=w1474) -> (x-y=w1473:i16)
            "BI Relative phase (D)" <- w1473
            n796 = feedback-in #67(w1473) -> ()
            n797 = feedback #69(TRUE) -> (w1484:bool)
            n798 = case shown="2" "Blue Laser Operating Mode (D)" {
              tunnel: [TRUE FALSE w1498] -> w1481
              tunnel: w1484 -> [_ _ w1495]
              frame 0, Default {
              }
              frame 1 {
              }
              frame 2 {
                n799 = Not(x=w1495) -> (.not. x?=w1497:bool)
                n800 = Select(t=w1497, s="Invert BI (D)", f=w1495) -> (s? t:f=w1498:bool)
              }
            }
            n801 = Not(x=w1484) -> (.not. x?=w1480:bool)
            n802 = Select(t="Blue interlace ON count (D)", s=w1480, f="Blue interlace OFF count (D)") -> (s? t:f=w1486:u16)
            n803 = Subtract(x=w1486, y=w1465) -> (x-y=w1478:u16)
            n804 = Add(x=w1478, y=w1474) -> (x+y=w1472:u16)
            n805 = feedback-in #69(w1480) -> ()
          }
        }
      }
    }
    frame Enabled {
    }
  }
